vi "cursor window logic -- sygnal plot -- V3.vi"(4 "h. offset":dbl, 6 "CursIdx":i32, 7 "cursor window action":T3=enum."check", 8 "window":dbl=nan, 9 "center":dbl=nan, 10 "cursor window IN":refnum<vi>, 11 "cursor window init":T1={"left"=2378.60310421286, "right "=2421.6740576496672, "center"=2421.6740576496672, "window"=2421.6740576496672, "cursors"=[], "relative"=0, "absolute"=0, "fixed vertical offset"=2421.6740576496672, "vertical offset"=2421.6740576496672, "skew"=2421.6740576496672, "default window frac"=2421.6740576496672, "kind"=enum."skewed", "skew.left"=2421.6740576496672, "skew.right"=2421.6740576496672, "wing order"=enum."back", "Plot ref Syg"=refnum}) -> (2 "cursor window OUT":refnum<vi>, 3 "cursor window out":T1={"left"=2378.60310421286, "right "=2421.6740576496672, "center"=2421.6740576496672, "window"=2421.6740576496672, "cursors"=[], "relative"=0, "absolute"=0, "fixed vertical offset"=2421.6740576496672, "vertical offset"=2421.6740576496672, "skew"=2421.6740576496672, "default window frac"=2421.6740576496672, "kind"=enum."skewed", "skew.left"=2421.6740576496672, "skew.right"=2421.6740576496672, "wing order"=enum."back", "Plot ref Syg"=refnum})   [LabVIEW 2021]
uses:
  cursor window action.ctl
  cursor winow sygnal plot.ctl
  comparison control.ctl
  cursor window state.ctl
  stack action -- control.ctl
  cursor action.ctl
  2Dwindow-centerwin.ctl
  range multiplier action.ctl
  cursor sate.ctl
  replace cursor action stack.vi
  Q - not nan and gtr than zero - Real.vi
  Q - not nan -- real.vi
  array - smart min max.vi
  Q - not nan -- integer.vi
panel:
  in  "cursor window":T1={"left"=2378.60310421286, "right "=2421.6740576496672, "center"=2421.6740576496672, "window"=2421.6740576496672, "cursors"=[], "relative"=0, "absolute"=0, "fixed vertical offset"=2421.6740576496672, "vertical offset"=2421.6740576496672, "skew"=2421.6740576496672, "default window frac"=2421.6740576496672, "kind"=enum."skewed", "skew.left"=2421.6740576496672, "skew.right"=2421.6740576496672, "wing order"=enum."back", "Plot ref Syg"=refnum}
  out "Signal graph 2":waveform(dbl)[](graph)
  out "selector":T2
  out "result":bool
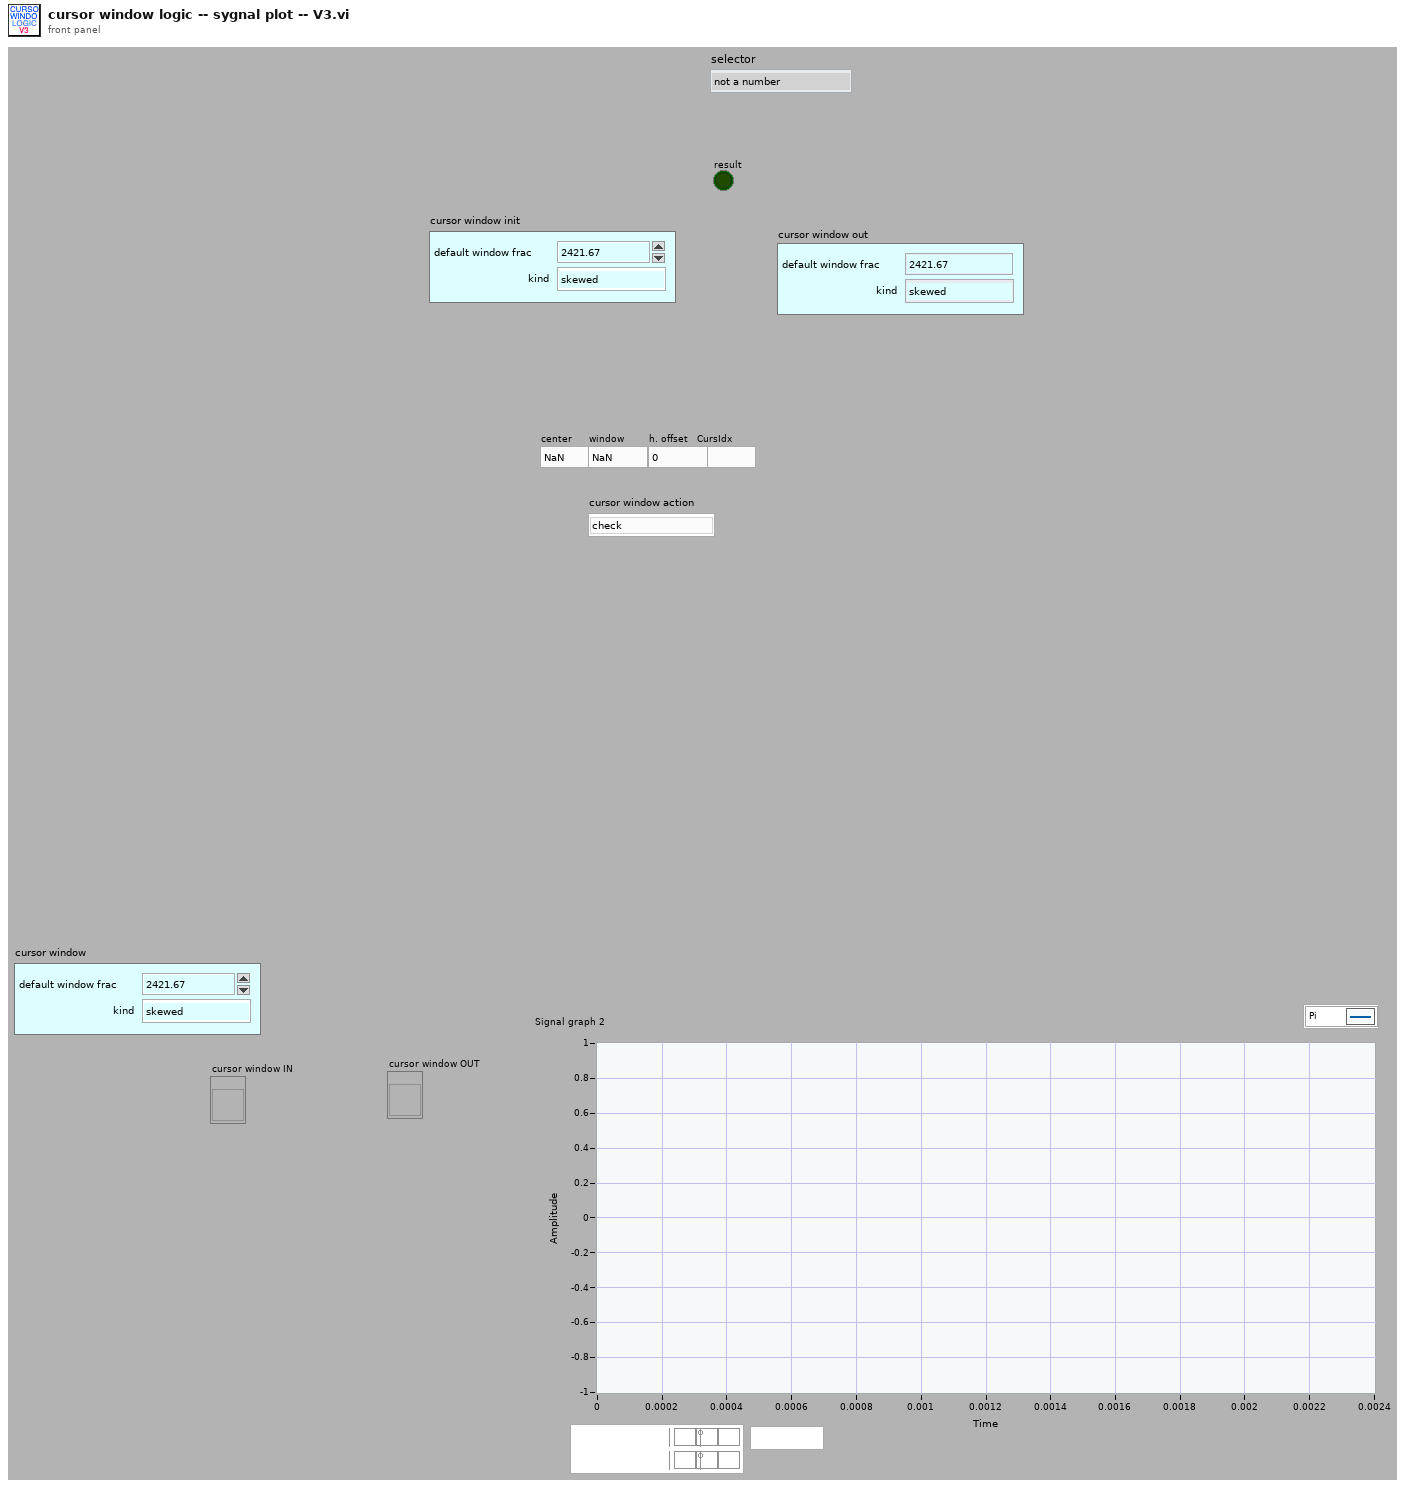
[diagram p1: front panel]
types:
  T1 = typedef "cursor winow sygnal plot.ctl" = cluster{"left":dbl, "right ":dbl, "center":dbl, "window":dbl, "cursors":i32[], "relative":i32, "absolute":i32, "fixed vertical offset":dbl, "vertical offset":dbl, "skew":dbl, "default window frac":dbl, "kind":enum16{"symmetric", "skewed", "fancy"}, "skew.left":dbl, "skew.right":dbl, "wing order":enum16{"forw", "back"}, "Plot ref Syg":refnum<vi>}
  T2 = typedef "comparison control.ctl" = enum16{"not a number", "above", "in range", "below"}
  T3 = typedef "cursor window action.ctl" = enum16{"balance", "h. offset change", "cursor moves", "change center", "change window", "init", "check", "reset", "set y to middle", "idle", "-write all Y", "-write left.X", "-write center.X", "-write right.X", "-write all X", "-change center", "-change window", "-change skew", "-read cursor 2", "-read cursor 1", "-read cursor 0", "-read all cursors", "-reset", "-read plot scale", "-set y to middle", "-Q: center.Y is visible", "-Q: window is visible", "-parse center.Y", "-right left from center", "-left move", "-right move", "-set center.Y", "-empty", "-set cursors to default", "-check", "-write center.Y", "-copy cursor 1", "-copy cursor 0", "-copy cursor 2", "move right", "move left", "shrink", "broaden", "skew up", "skew down", "-write plot scale", "zoom X", "change cen&win", "zoom to all data", "color--red", "color--green", "color--yellow", "read", "zoom out", "zoom in", "slide right", "slide left", "set range aspect ratio to 1", "move to window range", "--move to window range"}
  T4 = typedef "cursor window state.ctl" = cluster{"scale.y.halfwidth":dbl, "scale.y.center":dbl, "scale.x.halfwidth":dbl, "scale.x.center":dbl, "cursor":i32, "skew":dbl, "scale.y.max":dbl, "scale.x.range":dbl, "scale.y.min":dbl, "scale.y.range":dbl, "scale.x.min":dbl, "scale.x.max":dbl, "center.Y":dbl, "center.X":dbl, "left.Y":dbl, "left.X":dbl, "right.X":dbl, "right.Y":dbl}
  T5 = typedef "stack action -- control.ctl" = enum16{"push", "pop", "check", "init"}
  T6 = cluster{"center":dbl, "window":dbl, "h.offset":dbl, "cursor window":T1}
  T7 = typedef "cursor action.ctl" = enum16{"range", "read", "write", "check", "zoom out", "smart zoom out", "zoom to aspect ratio 1", "zoom to win", "zoom out 20%", "zoom in 20%", "-empty", "smart zoom out&aspect", "move range left 20%", "move range right 20%", "move range up 20%", "move range down 20%", "zoom to X win", "zoom to Y win", "zoom out X", "zoom out Y", "zoom in X", "zoom in Y", "check plot scale", "set plot color", "set Xlabel", "set Ylabel", "set cursor color", "setlength", "empty", "hide plot", "unhide plot", "checklngth", "extend +1 if short", "extend +n if short"}
  T8 = typedef "2Dwindow-centerwin.ctl" = cluster{"window y":dbl, "center x":dbl, "center y":dbl, "window x":dbl}
  T9 = typedef "range multiplier action.ctl" = enum16{"shift", "zoom", "check"}
  T10 = typedef "2Dwindow-bounds.ctl" = cluster{"min y":dbl, "max x":dbl, "min x":dbl, "max y":dbl}
  T11 = typedef "cursor sate.ctl" = enum16{"normal", "alert", "fuzzy", "interesting", "boring", "colored"}
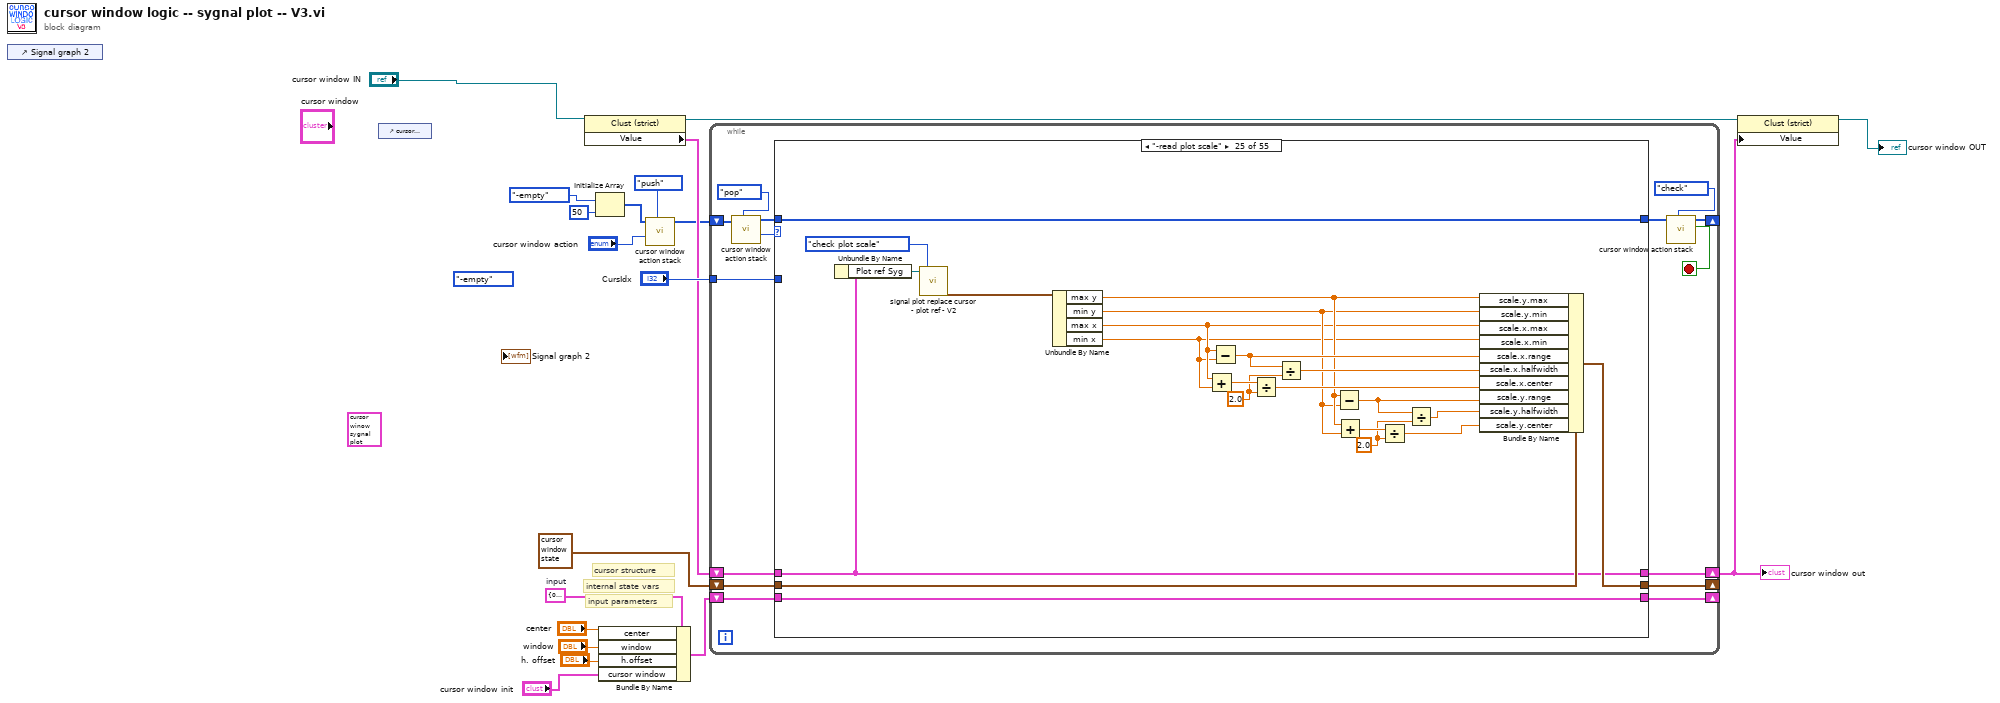
[diagram p0: block diagram]
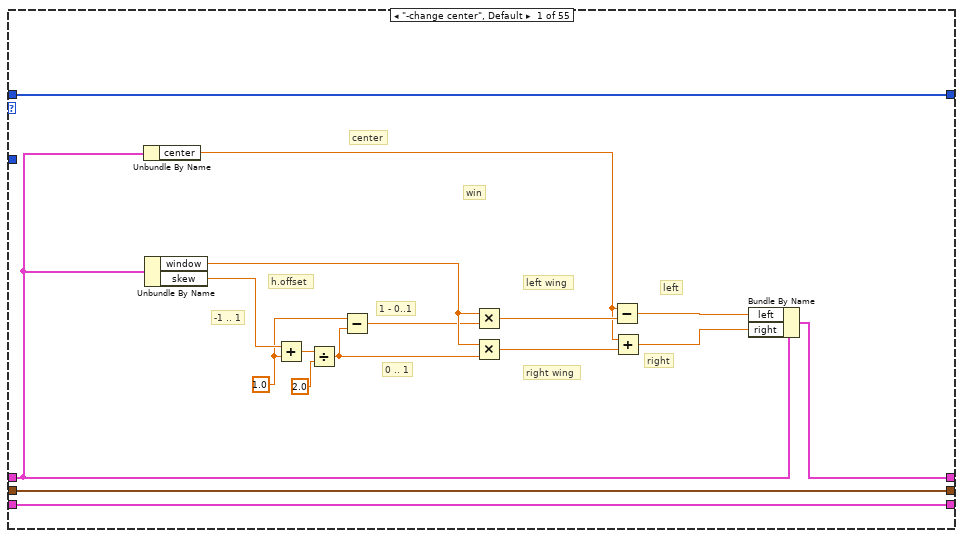
[diagram p2: hidden frame]
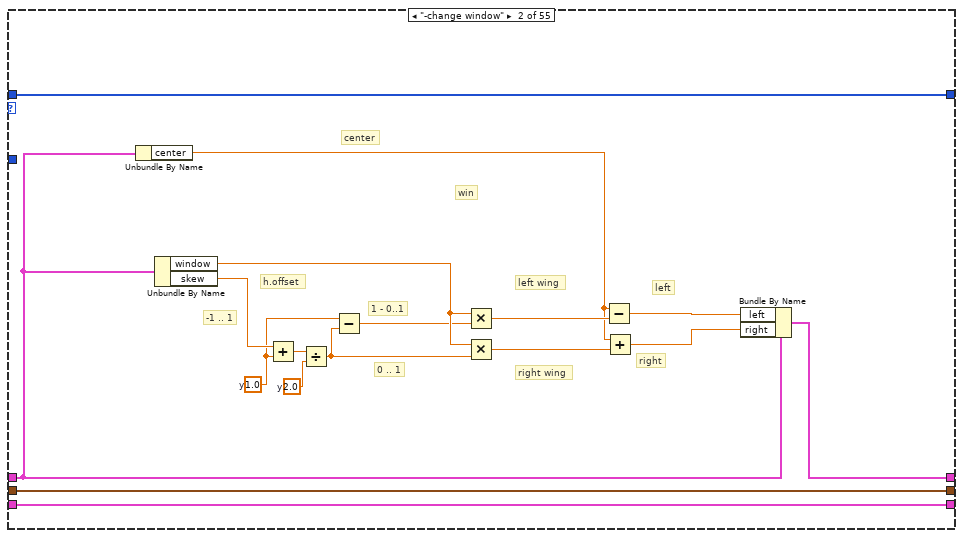
[diagram p3: hidden frame]
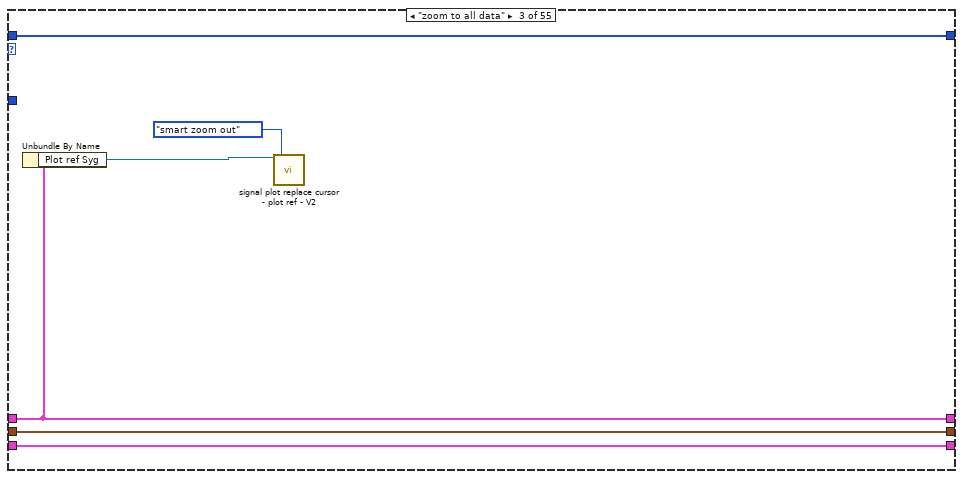
[diagram p4: hidden frame]
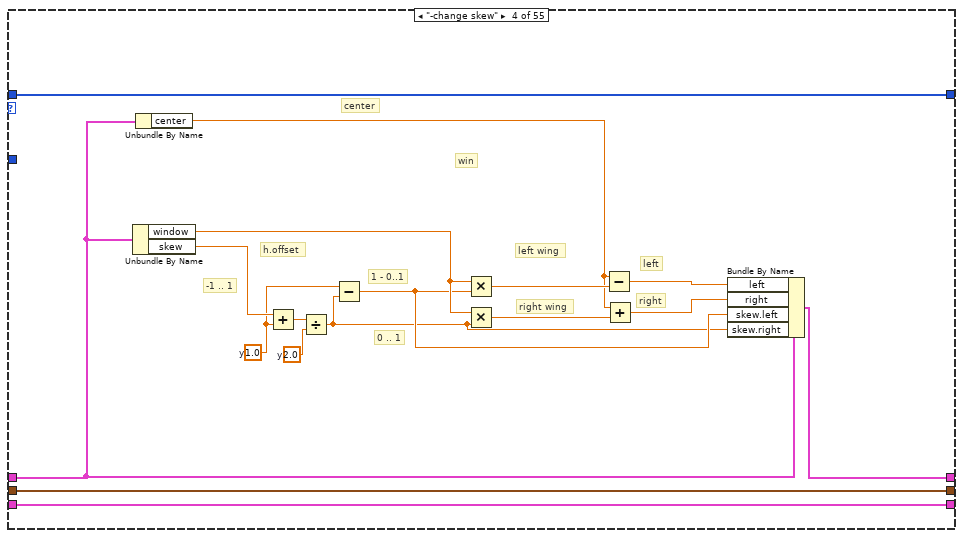
[diagram p5: hidden frame]
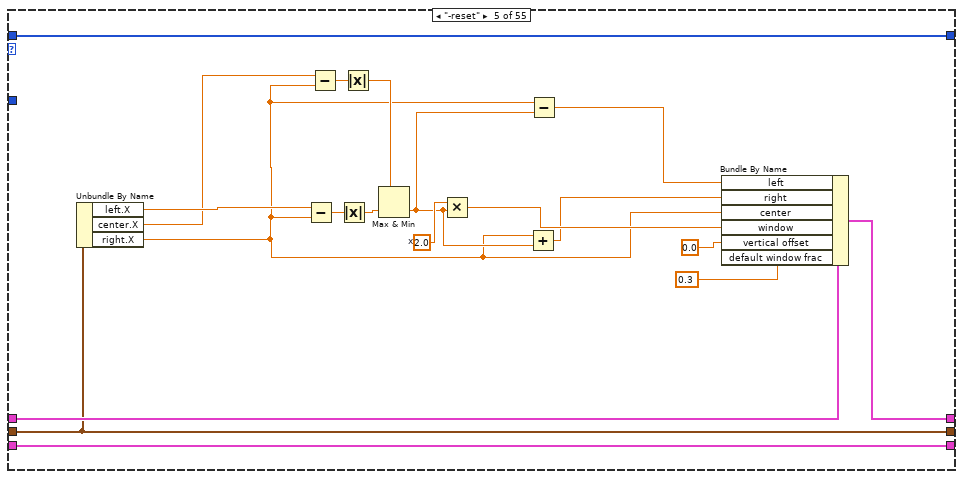
[diagram p6: hidden frame]
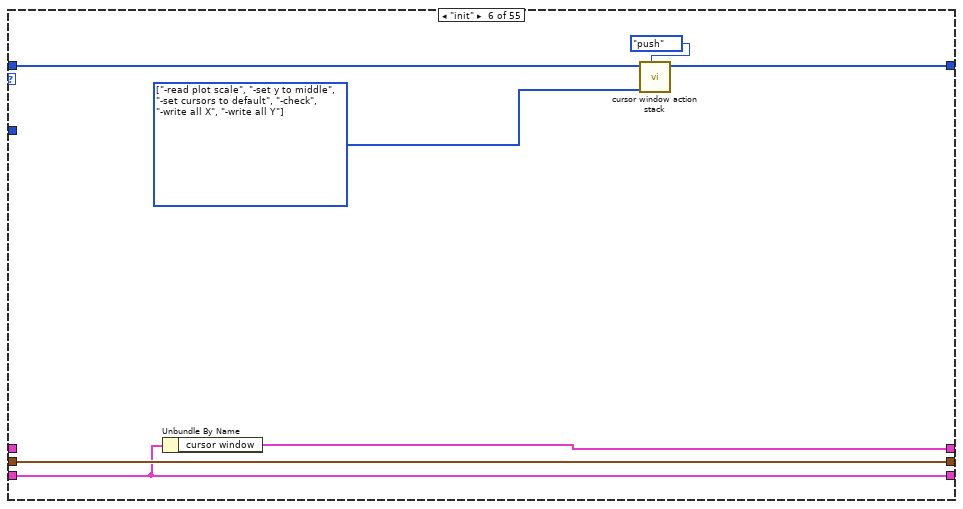
[diagram p7: hidden frame]
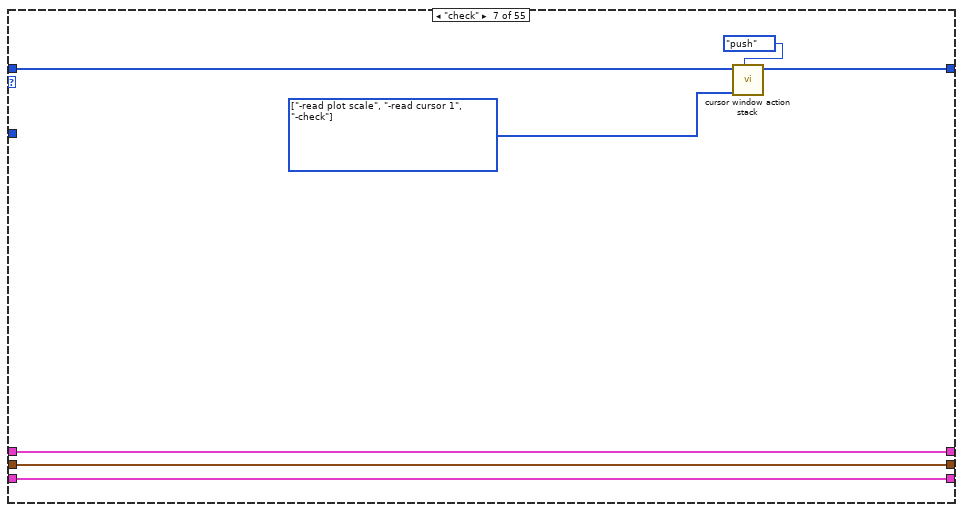
[diagram p8: hidden frame]
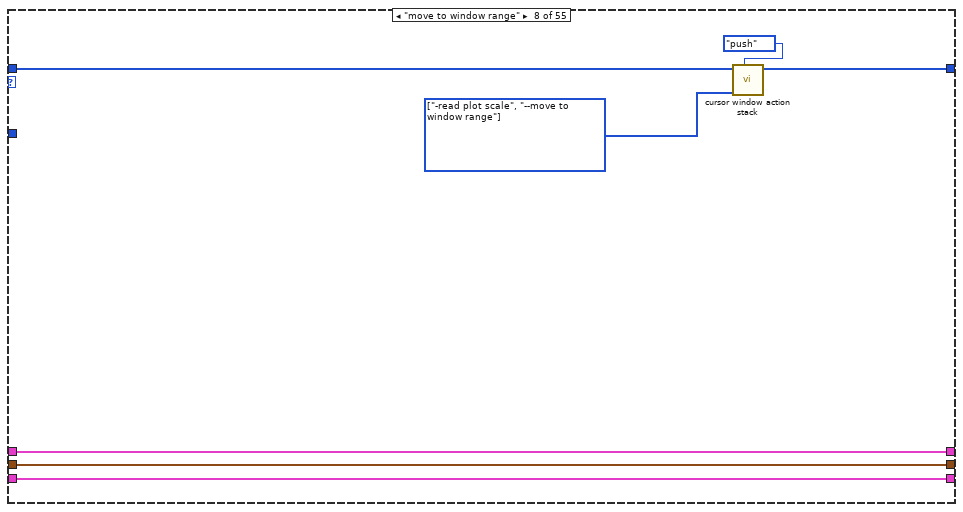
[diagram p9: hidden frame]
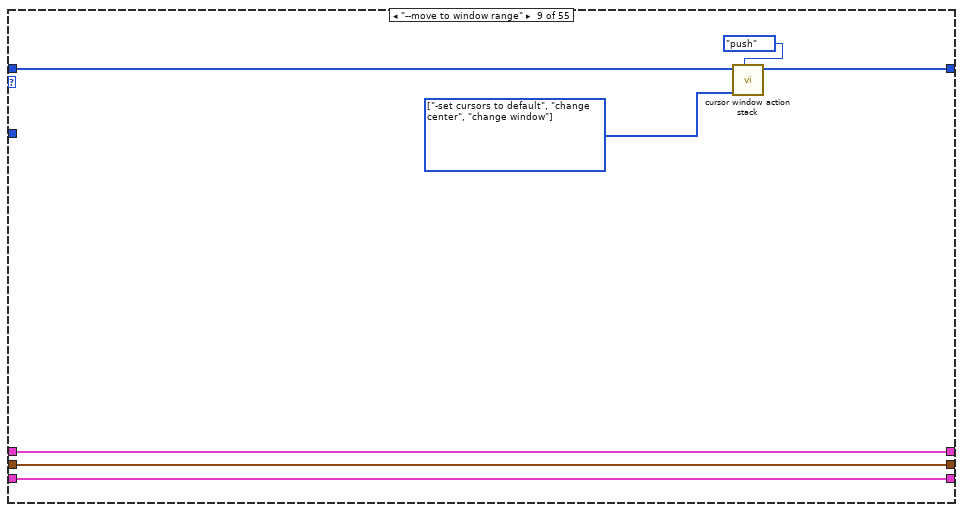
[diagram p10: hidden frame]
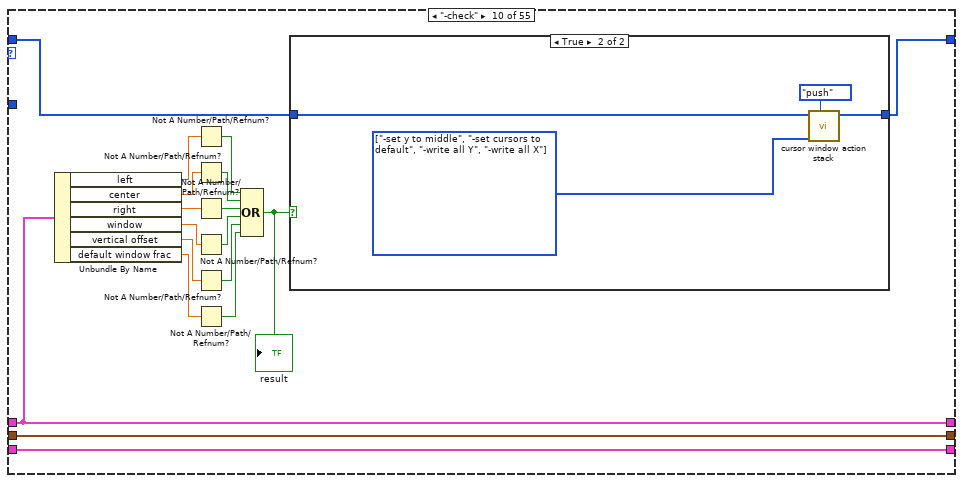
[diagram p11: hidden frame]
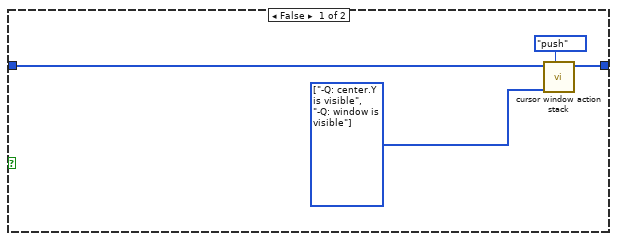
[diagram p12: hidden frame]
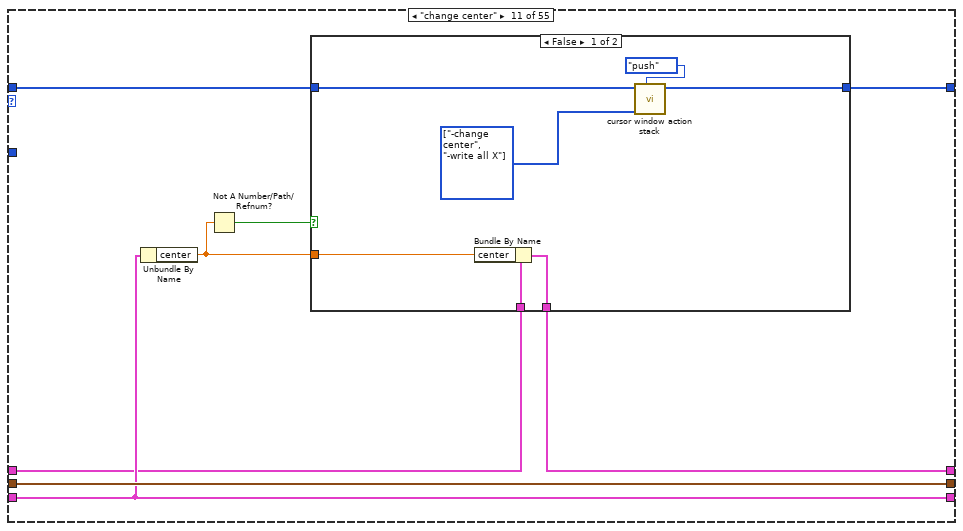
[diagram p13: hidden frame]
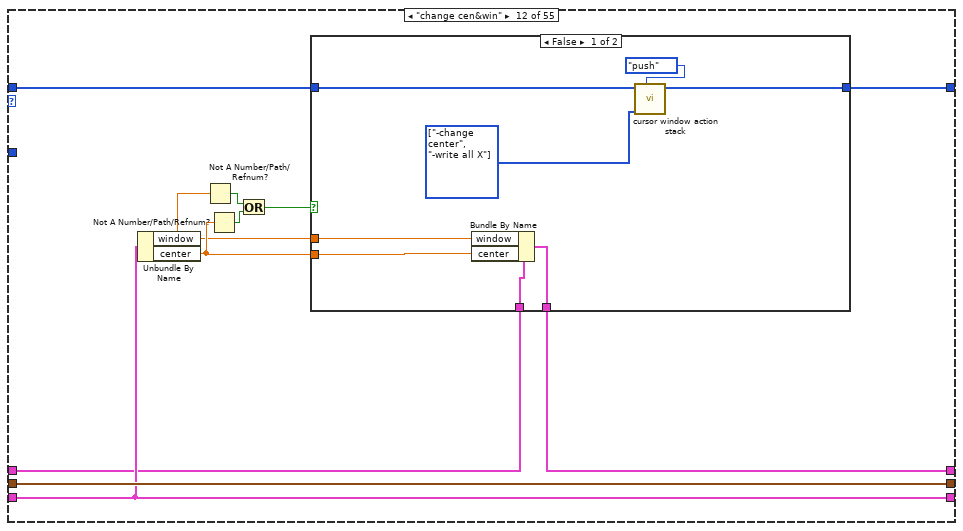
[diagram p15: hidden frame]
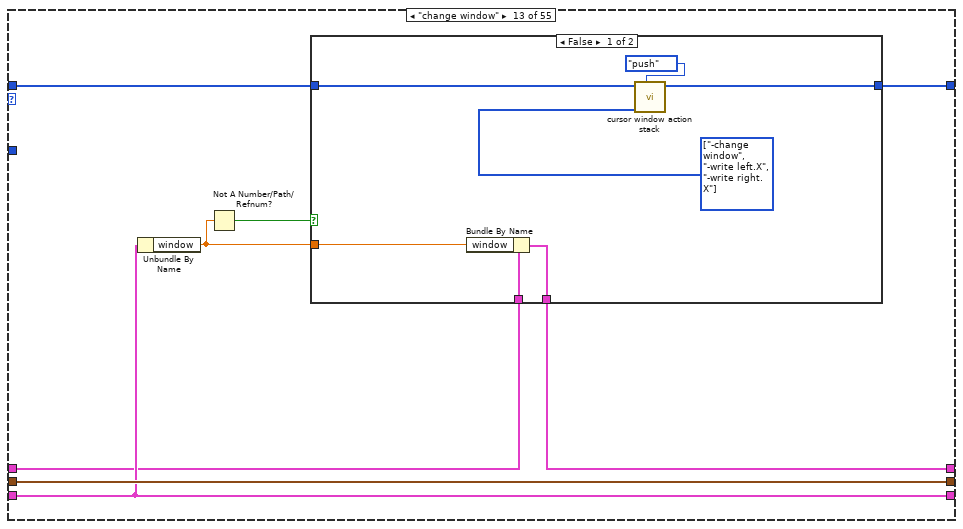
[diagram p17: hidden frame]
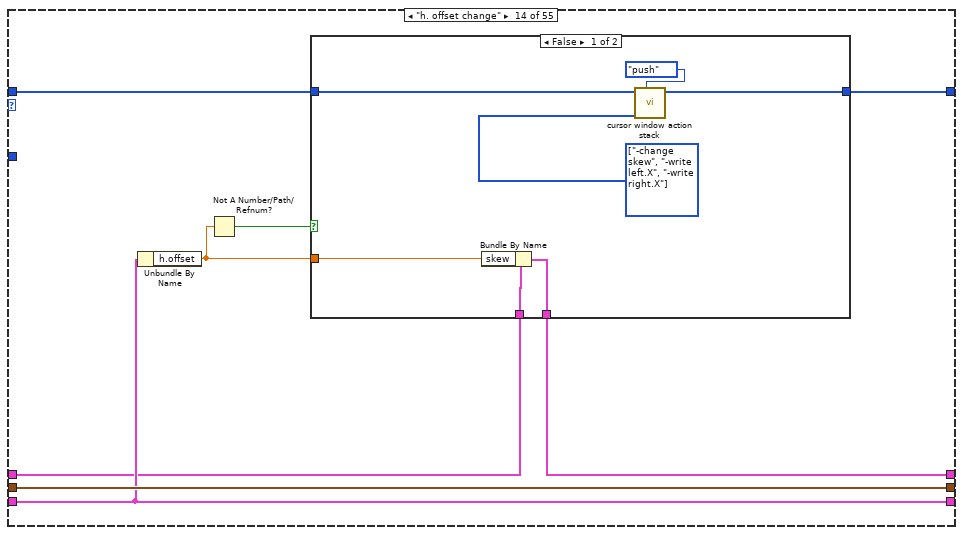
[diagram p19: hidden frame]
diagram:
  (unwired) T1 {"left"=2378.60310421286, "right "=2421.6740576496672, "center"=2421.6740576496672, "window"=2421.6740576496672, "cursors"=[], "relative"=0, "absolute"=0, "fixed vertical offset"=2421.6740576496672, "vertical offset"=2421.6740576496672, "skew"=2421.6740576496672, "default window frac"=2421.6740576496672, "kind"=enum."skewed", "skew.left"=2421.6740576496672, "skew.right"=2421.6740576496672, "wing order"=enum."back", "Plot ref Syg"=refnum} ("cursor window")
  (unwired) cursor_window_action."-empty" ("cursor window action")
  w18 = T6 {"center"=0.0, "window"=0.0, "h.offset"=0.0, "cursor window"={"left"=2378.60310421286, "right "=2421.6740576496672, "center"=2421.6740576496672, "window"=2421.6740576496672, "cursors"=[], "relative"=0, "absolute"=0, "fixed vertical offset"=2421.6740576496672, "vertical offset"=2421.6740576496672, "skew"=2421.6740576496672, "default window frac"=2421.6740576496672, "kind"=enum."skewed", "skew.left"=2421.6740576496672, "skew.right"=2421.6740576496672, "wing order"=enum."back", "Plot ref Syg"=refnum}}  # input
  # "input parameters"
  # "internal state vars"
  # "cursor structure"
  n1 = control-ref of="Signal graph 2"() -> ()  [unwired: 1 out]
  n2 = control-ref of="cursor window"() -> ()  [unwired: 1 out]
  n3 = property class="Clust (strict)"(reference="cursor window IN") -> (reference out=w19:refnum<vi>, "Value"=w12:T1)  [unwired: 1 in, 1 out]
  n4 = Initialize Array(cursor_window_action."-empty" ("cursor window action"), 50 ("dimension size")) -> (w7:T3[])
  n5 = Bundle By Name(cluster=w18, "center"="center", "window"="window", "h.offset"="h. offset", "cursor window"="cursor window init") -> (w14:T6)
  n6 = call "cursor window action stack.vi"("stack action"=stack_action_--_control."push", "cursor window action"="cursor window action", "command stack"=w7) -> ("command stack out"=w6:T3[])  [unwired: 6 in, 2 out]
  n7 = while {
    shift-right: [w27] -> _
    shift-left: w6 -> [w33]
    shift-right: [w20] -> w11
    shift-left: w12 -> [w34]
    shift-right: [w24] -> _
    shift-left: w14 -> [w25]
    shift-right: [w22] -> _
    shift-left: T4 {"scale.y.halfwidth"=nan, "scale.y.center"=nan, "scale.x.halfwidth"=nan, "scale.x.center"=nan, "cursor"=0, "skew"=nan, "scale.y.max"=nan, "scale.x.range"=nan, "scale.y.min"=nan, "scale.y.range"=nan, "scale.x.min"=nan, "scale.x.max"=nan, "center.Y"=nan, "center.X"=nan, "left.Y"=nan, "left.X"=nan, "right.X"=nan, "right.Y"=nan} ("state variables") -> [w23]
    tunnel: "CursIdx" -> [w21]
    stop <- w26 stop-if-true
    n8 = call "cursor window action stack.vi"("stack action"=stack_action_--_control."pop", "command stack"=w33) -> ("cursor window action out"=w32:T3, "command stack out"=w30:T3[])  [unwired: 7 in, 1 out]
    n9 = case shown="\"-read plot scale\"" w32 {
      tunnel: w34 -> [w36 w53 w71 w78 w100 _ w118 w125 w132 w142 w166 w187 w204 w221 w237 w244 w261 w295 w330 w369 w401 w405 w412 w431 w445 w471 w486 w492 w498 w504 w510 w516 w523 w547 w553 w573 w579 w592 w613 w652 w686 w726 w747 w767 w787 w808 w822 w839 w858 w871 w880 w903 w907 w920 w934]
      tunnel: [w40 w57 w74 w82 w99 w112 w121 w128 w135 w139 w171 w191 w209 w226 w240 w247 w258 w292 w332 w370 w402 w403 w421 w437 w456 w472 w487 w493 w499 w505 w511 w517 w521 w548 w561 w574 w588 w596 w617 w650 w688 w743 w763 w783 w803 w821 w836 w853 w867 w879 w901 w905 w919 w933 w947] -> w28
      tunnel: w30 -> [w40 w57 w74 w82 w99 w113 w122 w129 w136 w140 w170 w190 w208 w225 w241 w248 w258 w292 w332 w357 w402 w403 w421 w437 w456 w472 w487 w493 w499 w505 w511 w517 w522 w549 w562 w575 w589 w597 w618 w650 w689 w743 w763 w783 w803 w821 w836 w853 w867 w879 w901 w905 w919 w933 w947]
      tunnel: w25 -> [w37 w54 w72 w79 w98 w116 w119 w126 w133 w143 w169 w189 w207 w224 w243 w250 w260 w294 w331 w362 w399 w406 w420 w436 w459 w473 w488 w494 w500 w506 w512 w518 w529 w543 w559 w569 w586 w593 w614 w668 w693 w728 w749 w769 w789 w810 w828 w846 w860 w873 w882 w904 w909 w923 w937]
      tunnel: [w37 w54 w72 w79 w98 w116 w119 w126 w133 w143 w169 w189 w207 w224 w243 w250 w260 w294 w331 w362 w399 w406 w420 w436 w459 w473 w488 w494 w500 w506 w512 w518 w529 w543 w559 w569 w586 w593 w614 w668 w693 w728 w749 w769 w789 w810 w828 w846 w860 w873 w882 w904 w909 w923 w937] -> w24
      tunnel: w23 -> [w39 w56 w73 w81 w97 w117 w120 w127 w134 w144 w172 w192 w210 w227 w242 w249 w259 w293 w336 w363 w400 w408 w417 w435 w458 w470 w485 w491 w497 w503 w509 w515 w525 w544 w560 w570 w587 w594 w615 w656 w692 w729 w750 w770 w790 w807 w829 w847 w861 w870 w890 w902 w913 w927 w941]
      tunnel: [w39 w56 w73 w81 w97 w117 w120 w127 w134 w144 w172 w192 w210 w227 w242 w249 w259 w293 w335 w363 w400 w408 w416 w435 w457 w470 w485 w491 w497 w503 w509 w515 w524 w544 w560 w570 w587 w594 w615 w659 w692 w729 w750 w770 w790 w807 w829 w847 w861 w870 w889 w902 w912 w926 w940] -> w22
      tunnel: w21 -> [_ _ _ _ _ _ _ _ _ _ _ _ _ _ _ _ _ _ _ w360 _ _ _ _ _ _ _ _ _ _ _ _ _ _ _ _ _ _ _ _ _ _ _ _ _ _ _ _ _ _ _ _ _ _ _]
      tunnel: [w35 w52 w71 w77 w93 w111 w118 w125 w132 w142 w165 w186 w203 w220 w237 w244 w251 w285 w330 w361 w401 w404 w411 w427 w445 w471 w486 w492 w498 w504 w510 w516 w523 w546 w552 w572 w578 w595 w616 w648 w685 w726 w747 w767 w787 w808 w822 w839 w858 w871 w880 w903 w907 w920 w934] -> w20
      frame "-change center", Default {
        w45 = 1.0 ("y")
        # "1 - 0..1"
        # "right"
        # "left"
        # "win"
        # "h.offset"
        # "center"
        # "left wing"
        # "right wing"
        # "0 .. 1"
        # "-1 .. 1"
        n10 = Unbundle By Name(w36) -> ("center"=w38:dbl)
        n11 = Unbundle By Name(w36) -> ("window"=w50:dbl, "skew"=w51:dbl)
        n12 = Add(x=w51, y=w45) -> (x+y=w46:dbl)
        n13 = Divide(x=w46, y=2.0) -> (x/y=w42:dbl)
        n14 = Subtract(x=w45, y=w42) -> (x-y=w41:dbl)
        n15 = Multiply(x=w50, y=w41) -> (x*y=w44:dbl)
        n16 = Multiply(x=w50, y=w42) -> (x*y=w43:dbl)
        n17 = Subtract(x=w38, y=w44) -> (x-y=w49:dbl)
        n18 = Add(x=w38, y=w43) -> (x+y=w48:dbl)
        n19 = Bundle By Name(cluster=w36, "left"=w49, "right"=w48) -> (w35:T1)
      }
      frame "-change window" {
        w62 = 1.0  # y
        w64 = 2.0  # y
        # "1 - 0..1"
        # "right"
        # "left"
        # "win"
        # "h.offset"
        # "center"
        # "left wing"
        # "right wing"
        # "0 .. 1"
        # "-1 .. 1"
        n20 = Unbundle By Name(w53) -> ("center"=w55:dbl)
        n21 = Unbundle By Name(w53) -> ("window"=w67:dbl, "skew"=w68:dbl)
        n22 = Add(x=w68, y=w62) -> (x+y=w63:dbl)
        n23 = Divide(x=w63, y=w64) -> (x/y=w59:dbl)
        n24 = Subtract(x=w62, y=w59) -> (x-y=w58:dbl)
        n25 = Multiply(x=w67, y=w58) -> (x*y=w61:dbl)
        n26 = Multiply(x=w67, y=w59) -> (x*y=w60:dbl)
        n27 = Subtract(x=w55, y=w61) -> (x-y=w66:dbl)
        n28 = Add(x=w55, y=w60) -> (x+y=w65:dbl)
        n29 = Bundle By Name(cluster=w53, "left"=w66, "right"=w65) -> (w52:T1)
      }
      frame "zoom to all data" {
        n30 = Unbundle By Name(w71) -> ("Plot ref Syg"=w69:refnum<vi>)
        n31 = call "signal plot replace cursor - plot ref - V2.vi"("Signal graph IN"=w69, "cursor action"=cursor_action."smart zoom out") -> ()  [unwired: 14 in, 4 out]
      }
      frame "-change skew" {
        w85 = 1.0  # y
        w87 = 2.0  # y
        # "1 - 0..1"
        # "right"
        # "left"
        # "win"
        # "h.offset"
        # "center"
        # "left wing"
        # "right wing"
        # "0 .. 1"
        # "-1 .. 1"
        n32 = Unbundle By Name(w78) -> ("window"=w90:dbl, "skew"=w91:dbl)
        n33 = Unbundle By Name(w78) -> ("center"=w80:dbl)
        n34 = Add(x=w91, y=w85) -> (x+y=w86:dbl)
        n35 = Divide(x=w86, y=w87) -> (x/y=w75:dbl)
        n36 = Subtract(x=w85, y=w75) -> (x-y=w76:dbl)
        n37 = Multiply(x=w90, y=w76) -> (x*y=w84:dbl)
        n38 = Multiply(x=w90, y=w75) -> (x*y=w83:dbl)
        n39 = Subtract(x=w80, y=w84) -> (x-y=w89:dbl)
        n40 = Add(x=w80, y=w83) -> (x+y=w88:dbl)
        n41 = Bundle By Name(cluster=w78, "left"=w89, "right"=w88, "skew.left"=w76, "skew.right"=w75) -> (w77:T1)
      }
      frame "-reset" {
        w106 = 2.0  # x
        n42 = Unbundle By Name(w97) -> ("left.X"=w96:dbl, "center.X"=w94:dbl, "right.X"=w95:dbl)
        n43 = Subtract(x=w96, y=w95) -> (x-y=w109:dbl)
        n44 = Subtract(x=w94, y=w95) -> (x-y=w110:dbl)
        n45 = Absolute Value(x=w109) -> (abs(x)=w107:dbl)
        n46 = Absolute Value(x=w110) -> (abs(x)=w108:dbl)
        n47 = Max & Min(x=w108, y=w107) -> (min(x,y)=w104:dbl)  [unwired: 1 out]
        n48 = Multiply(x=w106, y=w104) -> (x*y=w105:dbl)
        n49 = Add(x=w95, y=w104) -> (x+y=w102:dbl)
        n50 = Subtract(x=w95, y=w104) -> (x-y=w103:dbl)
        n51 = Bundle By Name(cluster=w100, "left"=w103, "right"=w102, "center"=w95, "window"=w105, "vertical offset"=0.0, "default window frac"=0.3) -> (w93:T1)
      }
      frame "init" {
        w114 = T3[] [enum."-read plot scale", enum."-set y to middle", enum."-set cursors to default", enum."-check", enum."-write all X", enum."-write all Y"] items=["balance", "h. offset change", "cursor moves", "change center", "change window", "init", "check", "reset", "set y to middle", "idle", "-write all Y", "-write left.X", "-write center.X", "-write right.X", "-write all X", "-change center", "-change window", "-change skew", "-read cursor 2", "-read cursor 1", "-read cursor 0", "-read all cursors", "-reset", "-read plot scale", "-set y to middle", "-Q: center.Y is visible", "-Q: window is visible", "-parse center.Y", "-right left from center", "-left move", "-right move", "-set center.Y", "-empty", "-set cursors to default", "-check", "-write center.Y", "-copy cursor 1", "-copy cursor 0", "-copy cursor 2", "move right", "move left", "shrink", "broaden", "skew up", "skew down", "-write plot scale", "zoom X", "change cen&win", "zoom to all data", "color--red", "color--green", "color--yellow", "read", "zoom out", "zoom in", "slide right", "slide left", "set range aspect ratio to 1", "move to window range", "--move to window range"]
        n52 = Unbundle By Name(w116) -> ("cursor window"=w111:T1)
        n53 = call "cursor window action stack.vi"("stack action"=stack_action_--_control."push", "action list"=w114, "command stack"=w113) -> ("command stack out"=w112:T3[])  [unwired: 6 in, 2 out]
      }
      frame "check" {
        w123 = T3[] [enum."-read plot scale", enum."-read cursor 1", enum."-check"] items=["balance", "h. offset change", "cursor moves", "change center", "change window", "init", "check", "reset", "set y to middle", "idle", "-write all Y", "-write left.X", "-write center.X", "-write right.X", "-write all X", "-change center", "-change window", "-change skew", "-read cursor 2", "-read cursor 1", "-read cursor 0", "-read all cursors", "-reset", "-read plot scale", "-set y to middle", "-Q: center.Y is visible", "-Q: window is visible", "-parse center.Y", "-right left from center", "-left move", "-right move", "-set center.Y", "-empty", "-set cursors to default", "-check", "-write center.Y", "-copy cursor 1", "-copy cursor 0", "-copy cursor 2", "move right", "move left", "shrink", "broaden", "skew up", "skew down", "-write plot scale", "zoom X", "change cen&win", "zoom to all data", "color--red", "color--green", "color--yellow", "read", "zoom out", "zoom in", "slide right", "slide left", "set range aspect ratio to 1", "move to window range", "--move to window range"]
        n54 = call "cursor window action stack.vi"("stack action"=stack_action_--_control."push", "action list"=w123, "command stack"=w122) -> ("command stack out"=w121:T3[])  [unwired: 6 in, 2 out]
      }
      frame "move to window range" {
        w130 = T3[] [enum."-read plot scale", enum."--move to window range"] items=["balance", "h. offset change", "cursor moves", "change center", "change window", "init", "check", "reset", "set y to middle", "idle", "-write all Y", "-write left.X", "-write center.X", "-write right.X", "-write all X", "-change center", "-change window", "-change skew", "-read cursor 2", "-read cursor 1", "-read cursor 0", "-read all cursors", "-reset", "-read plot scale", "-set y to middle", "-Q: center.Y is visible", "-Q: window is visible", "-parse center.Y", "-right left from center", "-left move", "-right move", "-set center.Y", "-empty", "-set cursors to default", "-check", "-write center.Y", "-copy cursor 1", "-copy cursor 0", "-copy cursor 2", "move right", "move left", "shrink", "broaden", "skew up", "skew down", "-write plot scale", "zoom X", "change cen&win", "zoom to all data", "color--red", "color--green", "color--yellow", "read", "zoom out", "zoom in", "slide right", "slide left", "set range aspect ratio to 1", "move to window range", "--move to window range"]
        n55 = call "cursor window action stack.vi"("stack action"=stack_action_--_control."push", "action list"=w130, "command stack"=w129) -> ("command stack out"=w128:T3[])  [unwired: 6 in, 2 out]
      }
      frame "--move to window range" {
        w137 = T3[] [enum."-set cursors to default", enum."change center", enum."change window"] items=["balance", "h. offset change", "cursor moves", "change center", "change window", "init", "check", "reset", "set y to middle", "idle", "-write all Y", "-write left.X", "-write center.X", "-write right.X", "-write all X", "-change center", "-change window", "-change skew", "-read cursor 2", "-read cursor 1", "-read cursor 0", "-read all cursors", "-reset", "-read plot scale", "-set y to middle", "-Q: center.Y is visible", "-Q: window is visible", "-parse center.Y", "-right left from center", "-left move", "-right move", "-set center.Y", "-empty", "-set cursors to default", "-check", "-write center.Y", "-copy cursor 1", "-copy cursor 0", "-copy cursor 2", "move right", "move left", "shrink", "broaden", "skew up", "skew down", "-write plot scale", "zoom X", "change cen&win", "zoom to all data", "color--red", "color--green", "color--yellow", "read", "zoom out", "zoom in", "slide right", "slide left", "set range aspect ratio to 1", "move to window range", "--move to window range"]
        n56 = call "cursor window action stack.vi"("stack action"=stack_action_--_control."push", "action list"=w137, "command stack"=w136) -> ("command stack out"=w135:T3[])  [unwired: 6 in, 2 out]
      }
      frame "-check" {
        n57 = Unbundle By Name(w142) -> ("left"=w154:dbl, "center"=w153:dbl, "right"=w155:dbl, "window"=w156:dbl, "vertical offset"=w148:dbl, "default window frac"=w147:dbl)
        n58 = Not A Number/Path/Refnum?(number/path/refnum=w154) -> (NaN/Path/Refnum?=w152:bool)
        n59 = Not A Number/Path/Refnum?(number/path/refnum=w153) -> (NaN/Path/Refnum?=w151:bool)
        n60 = Not A Number/Path/Refnum?(number/path/refnum=w155) -> (NaN/Path/Refnum?=w150:bool)
        n61 = Not A Number/Path/Refnum?(number/path/refnum=w156) -> (NaN/Path/Refnum?=w149:bool)
        n62 = Not A Number/Path/Refnum?(number/path/refnum=w148) -> (NaN/Path/Refnum?=w145:bool)
        n63 = Not A Number/Path/Refnum?(number/path/refnum=w147) -> (NaN/Path/Refnum?=w146:bool)
        n64 = Compound Arithmetic op=OR(w152, w151, w150, w149, w145, w146) -> (w141:bool)
        "result" <- w141
        n65 = case shown="True" w141 {
          tunnel: w140 -> [w158 w162]
          tunnel: [w157 w161] -> w139
          frame False {
            w159 = T3[] [enum."-Q: center.Y is visible", enum."-Q: window is visible"] items=["balance", "h. offset change", "cursor moves", "change center", "change window", "init", "check", "reset", "set y to middle", "idle", "-write all Y", "-write left.X", "-write center.X", "-write right.X", "-write all X", "-change center", "-change window", "-change skew", "-read cursor 2", "-read cursor 1", "-read cursor 0", "-read all cursors", "-reset", "-read plot scale", "-set y to middle", "-Q: center.Y is visible", "-Q: window is visible", "-parse center.Y", "-right left from center", "-left move", "-right move", "-set center.Y", "-empty", "-set cursors to default", "-check", "-write center.Y", "-copy cursor 1", "-copy cursor 0", "-copy cursor 2", "move right", "move left", "shrink", "broaden", "skew up", "skew down", "-write plot scale", "zoom X", "change cen&win", "zoom to all data", "color--red", "color--green", "color--yellow", "read", "zoom out", "zoom in", "slide right", "slide left", "set range aspect ratio to 1", "move to window range", "--move to window range"]
            n66 = call "cursor window action stack.vi"("stack action"=stack_action_--_control."push", "action list"=w159, "command stack"=w158) -> ("command stack out"=w157:T3[])  [unwired: 6 in, 2 out]
          }
          frame True {
            w163 = T3[] [enum."-set y to middle", enum."-set cursors to default", enum."-write all Y", enum."-write all X"] items=["balance", "h. offset change", "cursor moves", "change center", "change window", "init", "check", "reset", "set y to middle", "idle", "-write all Y", "-write left.X", "-write center.X", "-write right.X", "-write all X", "-change center", "-change window", "-change skew", "-read cursor 2", "-read cursor 1", "-read cursor 0", "-read all cursors", "-reset", "-read plot scale", "-set y to middle", "-Q: center.Y is visible", "-Q: window is visible", "-parse center.Y", "-right left from center", "-left move", "-right move", "-set center.Y", "-empty", "-set cursors to default", "-check", "-write center.Y", "-copy cursor 1", "-copy cursor 0", "-copy cursor 2", "move right", "move left", "shrink", "broaden", "skew up", "skew down", "-write plot scale", "zoom X", "change cen&win", "zoom to all data", "color--red", "color--green", "color--yellow", "read", "zoom out", "zoom in", "slide right", "slide left", "set range aspect ratio to 1", "move to window range", "--move to window range"]
            n67 = call "cursor window action stack.vi"("stack action"=stack_action_--_control."push", "action list"=w163, "command stack"=w162) -> ("command stack out"=w161:T3[])  [unwired: 6 in, 2 out]
          }
        }
      }
      frame "change center" {
        n68 = Unbundle By Name(w169) -> ("center"=w167:dbl)
        n69 = Not A Number/Path/Refnum?(number/path/refnum=w167) -> (NaN/Path/Refnum?=w168:bool)
        n70 = case shown="False" w168 {
          tunnel: [w179 w180] -> w171
          tunnel: w170 -> [w178 w180]
          tunnel: w166 -> [w175 w181]
          tunnel: w167 -> [w174 _]
          tunnel: [w173 w181] -> w165
          frame False {
            w176 = T3[] [enum."-change center", enum."-write all X"] items=["balance", "h. offset change", "cursor moves", "change center", "change window", "init", "check", "reset", "set y to middle", "idle", "-write all Y", "-write left.X", "-write center.X", "-write right.X", "-write all X", "-change center", "-change window", "-change skew", "-read cursor 2", "-read cursor 1", "-read cursor 0", "-read all cursors", "-reset", "-read plot scale", "-set y to middle", "-Q: center.Y is visible", "-Q: window is visible", "-parse center.Y", "-right left from center", "-left move", "-right move", "-set center.Y", "-empty", "-set cursors to default", "-check", "-write center.Y", "-copy cursor 1", "-copy cursor 0", "-copy cursor 2", "move right", "move left", "shrink", "broaden", "skew up", "skew down", "-write plot scale", "zoom X", "change cen&win", "zoom to all data", "color--red", "color--green", "color--yellow", "read", "zoom out", "zoom in", "slide right", "slide left", "set range aspect ratio to 1", "move to window range", "--move to window range"]
            n71 = Bundle By Name(cluster=w175, "center"=w174) -> (w173:T1)
            n72 = call "cursor window action stack.vi"("stack action"=stack_action_--_control."push", "action list"=w176, "command stack"=w178) -> ("command stack out"=w179:T3[])  [unwired: 6 in, 2 out]
          }
          frame True {
          }
        }
      }
      frame "change cen&win" {
        n73 = Unbundle By Name(w189) -> ("window"=w182:dbl, "center"=w188:dbl)
        n74 = Not A Number/Path/Refnum?(number/path/refnum=w182) -> (NaN/Path/Refnum?=w185:bool)
        n75 = Not A Number/Path/Refnum?(number/path/refnum=w188) -> (NaN/Path/Refnum?=w184:bool)
        n76 = Or(x=w185, y=w184) -> (x .or. y?=w183:bool)
        n77 = case shown="False" w183 {
          tunnel: [w200 w201] -> w191
          tunnel: w190 -> [w199 w201]
          tunnel: w187 -> [w196 w202]
          tunnel: w188 -> [w195 _]
          tunnel: [w194 w202] -> w186
          tunnel: w182 -> [w193 _]
          frame False {
            w197 = T3[] [enum."-change center", enum."-write all X"] items=["balance", "h. offset change", "cursor moves", "change center", "change window", "init", "check", "reset", "set y to middle", "idle", "-write all Y", "-write left.X", "-write center.X", "-write right.X", "-write all X", "-change center", "-change window", "-change skew", "-read cursor 2", "-read cursor 1", "-read cursor 0", "-read all cursors", "-reset", "-read plot scale", "-set y to middle", "-Q: center.Y is visible", "-Q: window is visible", "-parse center.Y", "-right left from center", "-left move", "-right move", "-set center.Y", "-empty", "-set cursors to default", "-check", "-write center.Y", "-copy cursor 1", "-copy cursor 0", "-copy cursor 2", "move right", "move left", "shrink", "broaden", "skew up", "skew down", "-write plot scale", "zoom X", "change cen&win", "zoom to all data", "color--red", "color--green", "color--yellow", "read", "zoom out", "zoom in", "slide right", "slide left", "set range aspect ratio to 1", "move to window range", "--move to window range"]
            n78 = Bundle By Name(cluster=w196, "window"=w193, "center"=w195) -> (w194:T1)
            n79 = call "cursor window action stack.vi"("stack action"=stack_action_--_control."push", "action list"=w197, "command stack"=w199) -> ("command stack out"=w200:T3[])  [unwired: 6 in, 2 out]
          }
          frame True {
          }
        }
      }
      frame "change window" {
        n80 = Unbundle By Name(w207) -> ("window"=w205:dbl)
        n81 = Not A Number/Path/Refnum?(number/path/refnum=w205) -> (NaN/Path/Refnum?=w206:bool)
        n82 = case shown="False" w206 {
          tunnel: [w217 w218] -> w209
          tunnel: w208 -> [w216 w218]
          tunnel: w204 -> [w213 w219]
          tunnel: w205 -> [w212 _]
          tunnel: [w211 w219] -> w203
          frame False {
            w214 = T3[] [enum."-change window", enum."-write left.X", enum."-write right.X"] items=["balance", "h. offset change", "cursor moves", "change center", "change window", "init", "check", "reset", "set y to middle", "idle", "-write all Y", "-write left.X", "-write center.X", "-write right.X", "-write all X", "-change center", "-change window", "-change skew", "-read cursor 2", "-read cursor 1", "-read cursor 0", "-read all cursors", "-reset", "-read plot scale", "-set y to middle", "-Q: center.Y is visible", "-Q: window is visible", "-parse center.Y", "-right left from center", "-left move", "-right move", "-set center.Y", "-empty", "-set cursors to default", "-check", "-write center.Y", "-copy cursor 1", "-copy cursor 0", "-copy cursor 2", "move right", "move left", "shrink", "broaden", "skew up", "skew down", "-write plot scale", "zoom X", "change cen&win", "zoom to all data", "color--red", "color--green", "color--yellow", "read", "zoom out", "zoom in", "slide right", "slide left", "set range aspect ratio to 1", "move to window range", "--move to window range"]
            n83 = Bundle By Name(cluster=w213, "window"=w212) -> (w211:T1)
            n84 = call "cursor window action stack.vi"("stack action"=stack_action_--_control."push", "action list"=w214, "command stack"=w216) -> ("command stack out"=w217:T3[])  [unwired: 6 in, 2 out]
          }
          frame True {
          }
        }
      }
      frame "h. offset change" {
        n85 = Unbundle By Name(w224) -> ("h.offset"=w222:dbl)
        n86 = Not A Number/Path/Refnum?(number/path/refnum=w222) -> (NaN/Path/Refnum?=w223:bool)
        n87 = case shown="False" w223 {
          tunnel: [w234 w235] -> w226
          tunnel: w225 -> [w233 w235]
          tunnel: w221 -> [w230 w236]
          tunnel: w222 -> [w229 _]
          tunnel: [w228 w236] -> w220
          frame False {
            w231 = T3[] [enum."-change skew", enum."-write left.X", enum."-write right.X"] items=["balance", "h. offset change", "cursor moves", "change center", "change window", "init", "check", "reset", "set y to middle", "idle", "-write all Y", "-write left.X", "-write center.X", "-write right.X", "-write all X", "-change center", "-change window", "-change skew", "-read cursor 2", "-read cursor 1", "-read cursor 0", "-read all cursors", "-reset", "-read plot scale", "-set y to middle", "-Q: center.Y is visible", "-Q: window is visible", "-parse center.Y", "-right left from center", "-left move", "-right move", "-set center.Y", "-empty", "-set cursors to default", "-check", "-write center.Y", "-copy cursor 1", "-copy cursor 0", "-copy cursor 2", "move right", "move left", "shrink", "broaden", "skew up", "skew down", "-write plot scale", "zoom X", "change cen&win", "zoom to all data", "color--red", "color--green", "color--yellow", "read", "zoom out", "zoom in", "slide right", "slide left", "set range aspect ratio to 1", "move to window range", "--move to window range"]
            n88 = Bundle By Name(cluster=w230, "skew"=w229) -> (w228:T1)
            n89 = call "cursor window action stack.vi"("stack action"=stack_action_--_control."push", "action list"=w231, "command stack"=w233) -> ("command stack out"=w234:T3[])  [unwired: 6 in, 2 out]
          }
          frame True {
          }
        }
      }
      frame "reset" {
        w238 = T3[] [enum."-read plot scale", enum."-reset", enum."-write all X", enum."-write all Y"] items=["balance", "h. offset change", "cursor moves", "change center", "change window", "init", "check", "reset", "set y to middle", "idle", "-write all Y", "-write left.X", "-write center.X", "-write right.X", "-write all X", "-change center", "-change window", "-change skew", "-read cursor 2", "-read cursor 1", "-read cursor 0", "-read all cursors", "-reset", "-read plot scale", "-set y to middle", "-Q: center.Y is visible", "-Q: window is visible", "-parse center.Y", "-right left from center", "-left move", "-right move", "-set center.Y", "-empty", "-set cursors to default", "-check", "-write center.Y", "-copy cursor 1", "-copy cursor 0", "-copy cursor 2", "move right", "move left", "shrink", "broaden", "skew up", "skew down", "-write plot scale", "zoom X", "change cen&win", "zoom to all data", "color--red", "color--green", "color--yellow", "read", "zoom out", "zoom in", "slide right", "slide left", "set range aspect ratio to 1", "move to window range", "--move to window range"]
        n90 = call "cursor window action stack.vi"("stack action"=stack_action_--_control."push", "action list"=w238, "command stack"=w241) -> ("command stack out"=w240:T3[])  [unwired: 6 in, 2 out]
      }
      frame "set y to middle" {
        w245 = T3[] [enum."-read plot scale", enum."-set y to middle", enum."-write all Y"] items=["balance", "h. offset change", "cursor moves", "change center", "change window", "init", "check", "reset", "set y to middle", "idle", "-write all Y", "-write left.X", "-write center.X", "-write right.X", "-write all X", "-change center", "-change window", "-change skew", "-read cursor 2", "-read cursor 1", "-read cursor 0", "-read all cursors", "-reset", "-read plot scale", "-set y to middle", "-Q: center.Y is visible", "-Q: window is visible", "-parse center.Y", "-right left from center", "-left move", "-right move", "-set center.Y", "-empty", "-set cursors to default", "-check", "-write center.Y", "-copy cursor 1", "-copy cursor 0", "-copy cursor 2", "move right", "move left", "shrink", "broaden", "skew up", "skew down", "-write plot scale", "zoom X", "change cen&win", "zoom to all data", "color--red", "color--green", "color--yellow", "read", "zoom out", "zoom in", "slide right", "slide left", "set range aspect ratio to 1", "move to window range", "--move to window range"]
        n91 = call "cursor window action stack.vi"("stack action"=stack_action_--_control."push", "action list"=w245, "command stack"=w248) -> ("command stack out"=w247:T3[])  [unwired: 6 in, 2 out]
      }
      frame "-left move" {
        n92 = Unbundle By Name(w261) -> ("center"=w254:dbl, "skew.left"=w257:dbl, "skew.right"=w256:dbl)
        n93 = Unbundle By Name(w259) -> ("left.X"=w255:dbl)
        n94 = call "Q -- check range -- i -- real.vi"("upper"=w254, "number"=w255) -> ("selector"=w253:T2)  [unwired: 7 in, 2 out]
        n95 = case shown="\"in range\", Default" w253 {
          tunnel: w255 -> [w266 w284]
          tunnel: w256 -> [w272 w283]
          tunnel: [w273 w282] -> w262
          tunnel: [w268 w277] -> w264
          tunnel: w257 -> [w274 w281]
          tunnel: [w270 w276] -> w263
          tunnel: w254 -> [w267 w280]
          tunnel: [enum16{"forw", "back"}."forw" ("wing order") enum16{"forw", "back"}."back" ("wing order")] -> w252
          frame "in range", Default {
            # "right wing"
            # "left wing"
            n96 = Subtract(x=w267, y=w266) -> (x-y=w271:dbl)
            n97 = Divide(x=w271, y=w274) -> (x/y=w273:dbl)
            n98 = Multiply(x=w273, y=w272) -> (x*y=w269:dbl)
            n99 = Subtract(x=w267, y=w271) -> (x-y=w270:dbl)
            n100 = Add(x=w269, y=w267) -> (x+y=w268:dbl)
          }
          frame "above" {
            # "right wing"
            # "left wing"
            n101 = Subtract(x=w284, y=w280) -> (x-y=w279:dbl)
            n102 = Divide(x=w279, y=w283) -> (x/y=w282:dbl)
            n103 = Multiply(x=w282, y=w281) -> (x*y=w278:dbl)
            n104 = Subtract(x=w280, y=w278) -> (x-y=w276:dbl)
            n105 = Add(x=w279, y=w280) -> (x+y=w277:dbl)
          }
        }
        n106 = Bundle By Name(cluster=w261, "left"=w263, "right"=w264, "window"=w262, "wing order"=w252) -> (w251:T1)
      }
      frame "-right move" {
        n107 = Unbundle By Name(w295) -> ("center"=w286:dbl, "skew.left"=w291:dbl, "skew.right"=w290:dbl)
        n108 = Unbundle By Name(w293) -> ("right.X"=w289:dbl)
        n109 = call "Q -- check range -- i -- real.vi"("lower"=w286, "number"=w289) -> ("selector"=w288:T2)  [unwired: 7 in, 2 out]
        n110 = case shown="\"below\"" w288 {
          tunnel: w289 -> [w308 w310]
          tunnel: w290 -> [w307 w316]
          tunnel: [w306 w317] -> w296
          tunnel: [w301 w312] -> w298
          tunnel: w291 -> [w305 w318]
          tunnel: [w300 w314] -> w297
          tunnel: w286 -> [w304 w311]
          tunnel: [enum16{"forw", "back"}."forw" ("wing order") enum16{"forw", "back"}."back" ("wing order")] -> w287
          frame "in range", Default {
            # "right wing"
            n111 = Subtract(x=w308, y=w304) -> (x-y=w303:dbl)
            n112 = Divide(x=w303, y=w307) -> (x/y=w306:dbl)
            n113 = Multiply(x=w306, y=w305) -> (x*y=w302:dbl)
            n114 = Subtract(x=w304, y=w302) -> (x-y=w300:dbl)
            n115 = Add(x=w303, y=w304) -> (x+y=w301:dbl)
          }
          frame "below" {
            # "right wing"
            # "left wing"
            n116 = Subtract(x=w311, y=w310) -> (x-y=w315:dbl)
            n117 = Divide(x=w315, y=w318) -> (x/y=w317:dbl)
            n118 = Multiply(x=w317, y=w316) -> (x*y=w313:dbl)
            n119 = Subtract(x=w311, y=w315) -> (x-y=w314:dbl)
            n120 = Add(x=w313, y=w311) -> (x+y=w312:dbl)
          }
        }
        n121 = Bundle By Name(cluster=w295, "left"=w297, "right"=w298, "window"=w296, "wing order"=w287) -> (w285:T1)
      }
      frame "-set center.Y" {
        # "zero"
        # "calculate center.Y   from"
        # "complementary to calculation of fraction from vert offset"
        n122 = Unbundle By Name(w336) -> ("scale.y.halfwidth"=w333:dbl, "scale.y.center"=w334:dbl, "scale.x.range"=w340:dbl, "scale.y.max"=w339:dbl, "scale.y.min"=w338:dbl)
        n123 = Unbundle By Name(w330) -> ("window"=w341:dbl, "fixed vertical offset"=w342:dbl, "kind"=w320:enum16{"symmetric", "skewed", "fancy"}, "default window frac"=w343:dbl, "skew"=w319:dbl)
        n124 = case shown="\"symmetric\", Default" w320 {
          tunnel: w343 -> [w355 _]
          tunnel: w341 -> [w354 _]
          tunnel: w340 -> [w353 _]
          tunnel: [w344 w356] -> w321
          tunnel: w319 -> [_ w356]
          frame "symmetric", Default {
            # "window fraction"
            # "-1..1"
            n125 = Multiply(x=w353, y=w355) -> (x*y=w349:dbl)
            n126 = Divide(x=w354, y=w349) -> (x/y=w348:dbl)
            n127 = call "Q -- check range -- i -- real.vi"("upper"=0.99 ("y"), "lower"=0.0 ("y"), "number"=w348) -> ("number in range"=w345:dbl)  [unwired: 6 in, 2 out]
            n128 = Multiply(x=2.0, y=w345) -> (x*y=w352:dbl)
            n129 = Subtract(x=w352, y=1.0) -> (x-y=w344:dbl)
          }
          frame "skewed" {
          }
        }
        n130 = Multiply(x=w342, y=1.0) -> (x*y=w324:dbl)
        n131 = Multiply(x=w324, y=w333) -> (x*y=w329:dbl)
        n132 = Add(x=w334, y=w329) -> (x+y=w322:dbl)
        n133 = Subtract(x=w322, y=w338) -> (x-y=w327:dbl)
        n134 = Subtract(x=w339, y=w322) -> (x-y=w328:dbl)
        n135 = Max & Min(x=w328, y=w327) -> (min(x,y)=w326:dbl)  [unwired: 1 out]
        n136 = Multiply(x=w326, y=w321) -> (x*y=w323:dbl)
        n137 = Add(x=w322, y=w323) -> (x+y=w337:dbl)
        n138 = Bundle By Name(cluster=w336, "center.Y"=w337) -> (w335:T4)
      }
      frame "cursor moves" {
        n139 = Unbundle By Name(w369) -> ("cursors"=w368:i32[], "kind"=w359:enum16{"symmetric", "skewed", "fancy"})
        n140 = case shown="\"symmetric\", Default" w359 {
          tunnel: [w371 w375] -> w358
          tunnel: w357 -> [w371 w374]
          frame "symmetric", Default {
          }
          frame "fancy" {
            n141 = call "cursor window action stack.vi"("stack action"=stack_action_--_control."push", "cursor window action"=cursor_window_action."-write plot scale", "command stack"=w374) -> ("command stack out"=w375:T3[])  [unwired: 6 in, 2 out]
          }
        }
        n142 = Array Max & Min(array=w368) -> (max value=w366:i32, min value=w365:i32)  [unwired: 2 out]
        n143 = call "Q -- check range -- i -- integer.vi"("upper"=w366, "lower"=w365, "number"=w360) -> ("in range?"=w364:bool)  [unwired: 6 in, 2 out]
        n144 = Subtract(x=w360, y=w365) -> (x-y=w367:i32)
        n145 = case shown="True" w364 {
          tunnel: w358 -> [w377 w384]
          tunnel: [w377 w383] -> w370
          tunnel: w369 -> [w376 w382]
          tunnel: [w376 w381] -> w361
          tunnel: w368 -> [_ w380]
          tunnel: w367 -> [_ w379]
          frame False {
          }
          frame True {
            n146 = Index Array(array=w380, index=w379) -> (element=w378:i32)
            n147 = Bundle By Name(cluster=w382, "absolute"=w378, "relative"=w379) -> (w381:T1)
            n148 = case shown="0, 2, Default" w379 {
              selector: w379 -> [_ w394]
              tunnel: w384 -> [w388 w396]
              tunnel: [w387 w395] -> w383
              frame 1 {
                w385 = T3[] [enum."-read cursor 1", enum."-read plot scale", enum."-parse center.Y", enum."-copy cursor 1", enum."-change center", enum."-write right.X", enum."-write left.X"] items=["balance", "h. offset change", "cursor moves", "change center", "change window", "init", "check", "reset", "set y to middle", "idle", "-write all Y", "-write left.X", "-write center.X", "-write right.X", "-write all X", "-change center", "-change window", "-change skew", "-read cursor 2", "-read cursor 1", "-read cursor 0", "-read all cursors", "-reset", "-read plot scale", "-set y to middle", "-Q: center.Y is visible", "-Q: window is visible", "-parse center.Y", "-right left from center", "-left move", "-right move", "-set center.Y", "-empty", "-set cursors to default", "-check", "-write center.Y", "-copy cursor 1", "-copy cursor 0", "-copy cursor 2", "move right", "move left", "shrink", "broaden", "skew up", "skew down", "-write plot scale", "zoom X", "change cen&win", "zoom to all data", "color--red", "color--green", "color--yellow", "read", "zoom out", "zoom in", "slide right", "slide left", "set range aspect ratio to 1", "move to window range", "--move to window range"]
                n149 = call "cursor window action stack.vi"("stack action"=stack_action_--_control."push", "action list"=w385, "command stack"=w388) -> ("command stack out"=w387:T3[])  [unwired: 6 in, 2 out]
              }
              frame 0, 2, Default {
                w393 = T3[] [enum."-set center.Y", enum."-write center.Y"] items=["balance", "h. offset change", "cursor moves", "change center", "change window", "init", "check", "reset", "set y to middle", "idle", "-write all Y", "-write left.X", "-write center.X", "-write right.X", "-write all X", "-change center", "-change window", "-change skew", "-read cursor 2", "-read cursor 1", "-read cursor 0", "-read all cursors", "-reset", "-read plot scale", "-set y to middle", "-Q: center.Y is visible", "-Q: window is visible", "-parse center.Y", "-right left from center", "-left move", "-right move", "-set center.Y", "-empty", "-set cursors to default", "-check", "-write center.Y", "-copy cursor 1", "-copy cursor 0", "-copy cursor 2", "move right", "move left", "shrink", "broaden", "skew up", "skew down", "-write plot scale", "zoom X", "change cen&win", "zoom to all data", "color--red", "color--green", "color--yellow", "read", "zoom out", "zoom in", "slide right", "slide left", "set range aspect ratio to 1", "move to window range", "--move to window range"]
                w391 = T3[] [enum."-read plot scale"] items=["balance", "h. offset change", "cursor moves", "change center", "change window", "init", "check", "reset", "set y to middle", "idle", "-write all Y", "-write left.X", "-write center.X", "-write right.X", "-write all X", "-change center", "-change window", "-change skew", "-read cursor 2", "-read cursor 1", "-read cursor 0", "-read all cursors", "-reset", "-read plot scale", "-set y to middle", "-Q: center.Y is visible", "-Q: window is visible", "-parse center.Y", "-right left from center", "-left move", "-right move", "-set center.Y", "-empty", "-set cursors to default", "-check", "-write center.Y", "-copy cursor 1", "-copy cursor 0", "-copy cursor 2", "move right", "move left", "shrink", "broaden", "skew up", "skew down", "-write plot scale", "zoom X", "change cen&win", "zoom to all data", "color--red", "color--green", "color--yellow", "read", "zoom out", "zoom in", "slide right", "slide left", "set range aspect ratio to 1", "move to window range", "--move to window range"]
                n150 = case shown="0, Default" w394 {
                  tunnel: [w397 w398] -> w392
                  frame 0, Default {
                    w397 = T3[] [enum."-read cursor 0", enum."-left move", enum."-write right.X"] items=["balance", "h. offset change", "cursor moves", "change center", "change window", "init", "check", "reset", "set y to middle", "idle", "-write all Y", "-write left.X", "-write center.X", "-write right.X", "-write all X", "-change center", "-change window", "-change skew", "-read cursor 2", "-read cursor 1", "-read cursor 0", "-read all cursors", "-reset", "-read plot scale", "-set y to middle", "-Q: center.Y is visible", "-Q: window is visible", "-parse center.Y", "-right left from center", "-left move", "-right move", "-set center.Y", "-empty", "-set cursors to default", "-check", "-write center.Y", "-copy cursor 1", "-copy cursor 0", "-copy cursor 2", "move right", "move left", "shrink", "broaden", "skew up", "skew down", "-write plot scale", "zoom X", "change cen&win", "zoom to all data", "color--red", "color--green", "color--yellow", "read", "zoom out", "zoom in", "slide right", "slide left", "set range aspect ratio to 1", "move to window range", "--move to window range"]
                  }
                  frame 2 {
                    w398 = T3[] [enum."-read cursor 2", enum."-right move", enum."-write left.X"] items=["balance", "h. offset change", "cursor moves", "change center", "change window", "init", "check", "reset", "set y to middle", "idle", "-write all Y", "-write left.X", "-write center.X", "-write right.X", "-write all X", "-change center", "-change window", "-change skew", "-read cursor 2", "-read cursor 1", "-read cursor 0", "-read all cursors", "-reset", "-read plot scale", "-set y to middle", "-Q: center.Y is visible", "-Q: window is visible", "-parse center.Y", "-right left from center", "-left move", "-right move", "-set center.Y", "-empty", "-set cursors to default", "-check", "-write center.Y", "-copy cursor 1", "-copy cursor 0", "-copy cursor 2", "move right", "move left", "shrink", "broaden", "skew up", "skew down", "-write plot scale", "zoom X", "change cen&win", "zoom to all data", "color--red", "color--green", "color--yellow", "read", "zoom out", "zoom in", "slide right", "slide left", "set range aspect ratio to 1", "move to window range", "--move to window range"]
                  }
                }
                n151 = Build Array (concatenate)(w391, w392, w393) -> (w389:T3[])
                n152 = call "cursor window action stack.vi"("stack action"=stack_action_--_control."push", "action list"=w389, "command stack"=w396) -> ("command stack out"=w395:T3[])  [unwired: 6 in, 2 out]
              }
            }
          }
        }
      }
      frame "idle" {
      }
      frame "-copy cursor 1" {
        n153 = Unbundle By Name(w408) -> ("center.X"=w407:dbl)
        n154 = Bundle By Name(cluster=w405, "center"=w407) -> (w404:T1)
      }
      frame "-set y to middle" {
        w409 = 0.5
        n155 = Unbundle By Name(w412) -> ("fixed vertical offset"=w418:dbl)
        n156 = Unbundle By Name(w417) -> ("scale.y.center"=w413:dbl, "scale.y.halfwidth"=w414:dbl)
        n157 = Multiply(x=w414, y=w418) -> (x*y=w419:dbl)
        n158 = Bundle By Name(cluster=w412, "skew"=0.0, "skew.left"=w409, "skew.right"=w409) -> (w411:T1)
        n159 = Add(x=w413, y=w419) -> (x+y=w415:dbl)
        n160 = Bundle By Name(cluster=w417, "right.Y"=w415, "center.Y"=w415, "left.Y"=w415) -> (w416:T4)
      }
      frame "-set cursors to default" {
        w425 = 0.5
        w424 = 0.1
        (unwired) 3
        n161 = Unbundle By Name(w435) -> ("scale.x.halfwidth"=w423:dbl, "scale.x.center"=w429:dbl)
        n162 = Multiply(x=w423, y=w424) -> (x*y=w422:dbl)
        n163 = Multiply(x=w422, y=2) -> (x*y=w428:dbl)
        n164 = Add(x=w429, y=w422) -> (x+y=w433:dbl)
        n165 = Subtract(x=w429, y=w422) -> (x-y=w434:dbl)
        n166 = Bundle By Name(cluster=w431, "vertical offset"=0.0, "default window frac"=w424, "left"=w434, "right"=w433, "center"=w429, "window"=w428, "skew"=0.0, "skew.left"=w425, "skew.right"=w425) -> (w427:T1)
      }
      frame "-read plot scale" {
        w449 = 2.0 ("y")
        w454 = 2.0 ("y")
        n167 = Unbundle By Name(w445) -> ("Plot ref Syg"=w444:refnum<vi>)
        n168 = call "signal plot replace cursor - plot ref - V2.vi"("Signal graph IN"=w444, "cursor action"=cursor_action."check plot scale") -> ("2Dwindow bounds out"=w443:T10)  [unwired: 14 in, 3 out]
        n169 = Unbundle By Name(w443) -> ("max y"=w442:dbl, "min y"=w441:dbl, "max x"=w440:dbl, "min x"=w439:dbl)
        n170 = Add(x=w440, y=w439) -> (x+y=w455:dbl)
        n171 = Subtract(x=w440, y=w439) -> (x-y=w453:dbl)
        n172 = Divide(x=w455, y=w454) -> (x/y=w452:dbl)
        n173 = Divide(x=w453, y=w454) -> (x/y=w451:dbl)
        n174 = Subtract(x=w442, y=w441) -> (x-y=w446:dbl)
        n175 = Add(x=w442, y=w441) -> (x+y=w450:dbl)
        n176 = Divide(x=w450, y=w449) -> (x/y=w448:dbl)
        n177 = Divide(x=w446, y=w449) -> (x/y=w447:dbl)
        n178 = Bundle By Name(cluster=w458, "scale.y.max"=w442, "scale.y.min"=w441, "scale.x.max"=w440, "scale.x.min"=w439, "scale.x.range"=w453, "scale.x.halfwidth"=w451, "scale.x.center"=w452, "scale.y.range"=w446, "scale.y.halfwidth"=w447, "scale.y.center"=w448) -> (w457:T4)
      }
      frame "-write plot scale" {
        n179 = Unbundle By Name(w471) -> ("Plot ref Syg"=w464:refnum<vi>, "window"=w468:dbl, "center"=w467:dbl, "default window frac"=w466:dbl)
        n180 = call "Q -- range multiplier -- real -- V2.vi"("factor"=w466, "rage multiplier action"=range_multiplier_action."zoom", "center"=w467, "window"=w468) -> ("center OUT"=w462:dbl, "window OUT"=w461:dbl)  [unwired: 4 in, 2 out]
        n181 = Bundle By Name(cluster=T8 {"window y"=0.0021014740628288917, "center x"=44850.89441339177, "center y"=2.5658109925320947, "window x"=17480.201988350764} ("window IN"), "window x"=w461, "center x"=w462) -> (w460:T8)
        n182 = call "signal plot replace cursor - plot ref - V2.vi"("Signal graph IN"=w464, "window IN"=w460, "cursor action"=cursor_action."zoom to X win") -> ()  [unwired: 13 in, 4 out]
      }
      frame "zoom X" {
        n183 = Unbundle By Name(w486) -> ("Plot ref Syg"=w478:refnum<vi>, "window"=w477:dbl, "center"=w476:dbl, "default window frac"=w475:dbl)
        n184 = Reciprocal(x=w475) -> (1/x=w474:dbl)
        n185 = call "Q -- range multiplier -- real -- V2.vi"("factor"=w474, "rage multiplier action"=range_multiplier_action."zoom", "center"=w476, "window"=w477) -> ("center OUT"=w481:dbl, "window OUT"=w480:dbl)  [unwired: 4 in, 2 out]
        n186 = Bundle By Name(cluster=T8 {"window y"=0.0021014740628288917, "center x"=44850.89441339177, "center y"=2.5658109925320947, "window x"=17480.201988350764} ("window IN"), "window x"=w480, "center x"=w481) -> (w479:T8)
        n187 = call "signal plot replace cursor - plot ref - V2.vi"("Signal graph IN"=w478, "window IN"=w479, "cursor action"=cursor_action."zoom to X win") -> ()  [unwired: 13 in, 4 out]
      }
      frame "zoom out" {
        (unwired) range_multiplier_action."zoom" ("rage multiplier action")
        n188 = Unbundle By Name(w492) -> ("Plot ref Syg"=w489:refnum<vi>)
        n189 = call "signal plot replace cursor - plot ref - V2.vi"("Signal graph IN"=w489, "cursor action"=cursor_action."zoom out X") -> ()  [unwired: 14 in, 4 out]
      }
      frame "set range aspect ratio to 1" {
        n190 = Unbundle By Name(w498) -> ("Plot ref Syg"=w496:refnum<vi>)
        n191 = call "signal plot replace cursor - plot ref - V2.vi"("Signal graph IN"=w496, "cursor action"=cursor_action."zoom to aspect ratio 1") -> ()  [unwired: 14 in, 4 out]
      }
      frame "zoom in" {
        n192 = Unbundle By Name(w504) -> ("Plot ref Syg"=w502:refnum<vi>)
        n193 = call "signal plot replace cursor - plot ref - V2.vi"("Signal graph IN"=w502, "cursor action"=cursor_action."zoom in X") -> ()  [unwired: 14 in, 4 out]
      }
      frame "slide right" {
        n194 = Unbundle By Name(w510) -> ("Plot ref Syg"=w508:refnum<vi>)
        n195 = call "signal plot replace cursor - plot ref - V2.vi"("Signal graph IN"=w508, "cursor action"=cursor_action."move range right 20%") -> ()  [unwired: 14 in, 4 out]
      }
      frame "slide left" {
        n196 = Unbundle By Name(w516) -> ("Plot ref Syg"=w514:refnum<vi>)
        n197 = call "signal plot replace cursor - plot ref - V2.vi"("Signal graph IN"=w514, "cursor action"=cursor_action."move range left 20%") -> ()  [unwired: 14 in, 4 out]
      }
      frame "-Q: center.Y is visible" {
        # "check if y is within y-scale bounds"
        n198 = Unbundle By Name(w525) -> ("center.Y"=w528:dbl, "scale.y.max"=w527:dbl, "scale.y.min"=w526:dbl, "scale.y.center"=w519:dbl)
        n199 = call "Q -- check range -- i -- real.vi"("upper"=w527, "lower"=w526, "number"=w528) -> ("in range?"=w520:bool)  [unwired: 6 in, 2 out]
        n200 = case shown="False" w520 {
          tunnel: w525 -> [w536 w538]
          tunnel: [w535 w538] -> w524
          tunnel: w522 -> [w533 w537]
          tunnel: [w531 w537] -> w521
          tunnel: w519 -> [w530 _]
          frame False {
            w534 = T3[] [enum."-parse center.Y", enum."-write center.Y"] items=["balance", "h. offset change", "cursor moves", "change center", "change window", "init", "check", "reset", "set y to middle", "idle", "-write all Y", "-write left.X", "-write center.X", "-write right.X", "-write all X", "-change center", "-change window", "-change skew", "-read cursor 2", "-read cursor 1", "-read cursor 0", "-read all cursors", "-reset", "-read plot scale", "-set y to middle", "-Q: center.Y is visible", "-Q: window is visible", "-parse center.Y", "-right left from center", "-left move", "-right move", "-set center.Y", "-empty", "-set cursors to default", "-check", "-write center.Y", "-copy cursor 1", "-copy cursor 0", "-copy cursor 2", "move right", "move left", "shrink", "broaden", "skew up", "skew down", "-write plot scale", "zoom X", "change cen&win", "zoom to all data", "color--red", "color--green", "color--yellow", "read", "zoom out", "zoom in", "slide right", "slide left", "set range aspect ratio to 1", "move to window range", "--move to window range"]
            n201 = Bundle By Name(cluster=w536, "center.Y"=w530) -> (w535:T4)
            n202 = call "cursor window action stack.vi"("stack action"=stack_action_--_control."push", "action list"=w534, "command stack"=w533) -> ("command stack out"=w531:T3[])  [unwired: 6 in, 2 out]
          }
          frame True {
          }
        }
      }
      frame "move left" {
        (unwired) 0.2
        w551 = T3[] [enum."-change center", enum."-write all X"] items=["balance", "h. offset change", "cursor moves", "change center", "change window", "init", "check", "reset", "set y to middle", "idle", "-write all Y", "-write left.X", "-write center.X", "-write right.X", "-write all X", "-change center", "-change window", "-change skew", "-read cursor 2", "-read cursor 1", "-read cursor 0", "-read all cursors", "-reset", "-read plot scale", "-set y to middle", "-Q: center.Y is visible", "-Q: window is visible", "-parse center.Y", "-right left from center", "-left move", "-right move", "-set center.Y", "-empty", "-set cursors to default", "-check", "-write center.Y", "-copy cursor 1", "-copy cursor 0", "-copy cursor 2", "move right", "move left", "shrink", "broaden", "skew up", "skew down", "-write plot scale", "zoom X", "change cen&win", "zoom to all data", "color--red", "color--green", "color--yellow", "read", "zoom out", "zoom in", "slide right", "slide left", "set range aspect ratio to 1", "move to window range", "--move to window range"]
        n203 = Unbundle By Name(w547) -> ("center"=w541:dbl, "window"=w540:dbl, "default window frac"=w539:dbl)  [unwired: 1 out]
        n204 = Multiply(x=w540, y=w539) -> (x*y=w542:dbl)
        n205 = Subtract(x=w541, y=w542) -> (x-y=w545:dbl)
        n206 = Bundle By Name(cluster=w547, "center"=w545) -> (w546:T1)
        n207 = call "cursor window action stack.vi"("stack action"=stack_action_--_control."push", "action list"=w551, "command stack"=w549) -> ("command stack out"=w548:T3[])  [unwired: 6 in, 2 out]
      }
      frame "move right" {
        (unwired) 0.2
        w564 = T3[] [enum."-change center", enum."-write all X"] items=["balance", "h. offset change", "cursor moves", "change center", "change window", "init", "check", "reset", "set y to middle", "idle", "-write all Y", "-write left.X", "-write center.X", "-write right.X", "-write all X", "-change center", "-change window", "-change skew", "-read cursor 2", "-read cursor 1", "-read cursor 0", "-read all cursors", "-reset", "-read plot scale", "-set y to middle", "-Q: center.Y is visible", "-Q: window is visible", "-parse center.Y", "-right left from center", "-left move", "-right move", "-set center.Y", "-empty", "-set cursors to default", "-check", "-write center.Y", "-copy cursor 1", "-copy cursor 0", "-copy cursor 2", "move right", "move left", "shrink", "broaden", "skew up", "skew down", "-write plot scale", "zoom X", "change cen&win", "zoom to all data", "color--red", "color--green", "color--yellow", "read", "zoom out", "zoom in", "slide right", "slide left", "set range aspect ratio to 1", "move to window range", "--move to window range"]
        n208 = Unbundle By Name(w553) -> ("center"=w556:dbl, "window"=w555:dbl, "default window frac"=w554:dbl)  [unwired: 1 out]
        n209 = Multiply(x=w555, y=w554) -> (x*y=w557:dbl)
        n210 = Add(x=w556, y=w557) -> (x+y=w558:dbl)
        n211 = Bundle By Name(cluster=w553, "center"=w558) -> (w552:T1)
        n212 = call "cursor window action stack.vi"("stack action"=stack_action_--_control."push", "action list"=w564, "command stack"=w562) -> ("command stack out"=w561:T3[])  [unwired: 6 in, 2 out]
      }
      frame "shrink" {
        (unwired) 0.3
        w577 = T3[] [enum."-change window", enum."-write all X", enum."-read plot scale", enum."-set center.Y", enum."-write center.Y"] items=["balance", "h. offset change", "cursor moves", "change center", "change window", "init", "check", "reset", "set y to middle", "idle", "-write all Y", "-write left.X", "-write center.X", "-write right.X", "-write all X", "-change center", "-change window", "-change skew", "-read cursor 2", "-read cursor 1", "-read cursor 0", "-read all cursors", "-reset", "-read plot scale", "-set y to middle", "-Q: center.Y is visible", "-Q: window is visible", "-parse center.Y", "-right left from center", "-left move", "-right move", "-set center.Y", "-empty", "-set cursors to default", "-check", "-write center.Y", "-copy cursor 1", "-copy cursor 0", "-copy cursor 2", "move right", "move left", "shrink", "broaden", "skew up", "skew down", "-write plot scale", "zoom X", "change cen&win", "zoom to all data", "color--red", "color--green", "color--yellow", "read", "zoom out", "zoom in", "slide right", "slide left", "set range aspect ratio to 1", "move to window range", "--move to window range"]
        n213 = Unbundle By Name(w573) -> ("window"=w568:dbl, "window"=w567:dbl, "default window frac"=w565:dbl)
        n214 = Multiply(x=w567, y=w565) -> (x*y=w566:dbl)
        n215 = Subtract(x=w568, y=w566) -> (x-y=w571:dbl)
        n216 = Bundle By Name(cluster=w573, "window"=w571) -> (w572:T1)
        n217 = call "cursor window action stack.vi"("stack action"=stack_action_--_control."push", "action list"=w577, "command stack"=w575) -> ("command stack out"=w574:T3[])  [unwired: 6 in, 2 out]
      }
      frame "broaden" {
        (unwired) 0.3
        w585 = T3[] [enum."-change window", enum."-write all X", enum."-read plot scale", enum."-set center.Y", enum."-write center.Y"] items=["balance", "h. offset change", "cursor moves", "change center", "change window", "init", "check", "reset", "set y to middle", "idle", "-write all Y", "-write left.X", "-write center.X", "-write right.X", "-write all X", "-change center", "-change window", "-change skew", "-read cursor 2", "-read cursor 1", "-read cursor 0", "-read all cursors", "-reset", "-read plot scale", "-set y to middle", "-Q: center.Y is visible", "-Q: window is visible", "-parse center.Y", "-right left from center", "-left move", "-right move", "-set center.Y", "-empty", "-set cursors to default", "-check", "-write center.Y", "-copy cursor 1", "-copy cursor 0", "-copy cursor 2", "move right", "move left", "shrink", "broaden", "skew up", "skew down", "-write plot scale", "zoom X", "change cen&win", "zoom to all data", "color--red", "color--green", "color--yellow", "read", "zoom out", "zoom in", "slide right", "slide left", "set range aspect ratio to 1", "move to window range", "--move to window range"]
        n218 = Unbundle By Name(w579) -> ("window"=w583:dbl, "window"=w582:dbl, "default window frac"=w580:dbl)
        n219 = Multiply(x=w582, y=w580) -> (x*y=w581:dbl)
        n220 = Add(x=w583, y=w581) -> (x+y=w584:dbl)
        n221 = Bundle By Name(cluster=w579, "window"=w584) -> (w578:T1)
        n222 = call "cursor window action stack.vi"("stack action"=stack_action_--_control."push", "action list"=w585, "command stack"=w589) -> ("command stack out"=w588:T3[])  [unwired: 6 in, 2 out]
      }
      frame "skew up" {
        n223 = Unbundle By Name(w592) -> ("kind"=w591:enum16{"symmetric", "skewed", "fancy"})
        n224 = case shown="\"skewed\"" w591 {
          tunnel: w597 -> [w599 w609]
          tunnel: [w599 w608] -> w596
          tunnel: [w598 w607] -> w595
          tunnel: w592 -> [w598 w605]
          frame "symmetric", Default {
          }
          frame "skewed" {
            w611 = T3[] [enum."-change skew", enum."-read plot scale", enum."-set center.Y", enum."-write right.X", enum."-write left.X", enum."-write center.Y"] items=["balance", "h. offset change", "cursor moves", "change center", "change window", "init", "check", "reset", "set y to middle", "idle", "-write all Y", "-write left.X", "-write center.X", "-write right.X", "-write all X", "-change center", "-change window", "-change skew", "-read cursor 2", "-read cursor 1", "-read cursor 0", "-read all cursors", "-reset", "-read plot scale", "-set y to middle", "-Q: center.Y is visible", "-Q: window is visible", "-parse center.Y", "-right left from center", "-left move", "-right move", "-set center.Y", "-empty", "-set cursors to default", "-check", "-write center.Y", "-copy cursor 1", "-copy cursor 0", "-copy cursor 2", "move right", "move left", "shrink", "broaden", "skew up", "skew down", "-write plot scale", "zoom X", "change cen&win", "zoom to all data", "color--red", "color--green", "color--yellow", "read", "zoom out", "zoom in", "slide right", "slide left", "set range aspect ratio to 1", "move to window range", "--move to window range"]
            n225 = Unbundle By Name(w605) -> ("skew"=w606:dbl)
            n226 = Add(x=0.1, y=w606) -> (x+y=w603:dbl)
            n227 = call "Q -- check range -- i -- real.vi"("upper"=1, "lower"=-1, "number"=w603) -> ("number in range"=w600:dbl)  [unwired: 6 in, 2 out]
            n228 = Bundle By Name(cluster=w605, "skew"=w600) -> (w607:T1)
            n229 = call "cursor window action stack.vi"("stack action"=stack_action_--_control."push", "action list"=w611, "command stack"=w609) -> ("command stack out"=w608:T3[])  [unwired: 6 in, 2 out]
          }
        }
      }
      frame "skew down" {
        n230 = Unbundle By Name(w613) -> ("kind"=w612:enum16{"symmetric", "skewed", "fancy"})
        n231 = case shown="\"skewed\"" w612 {
          tunnel: w618 -> [w620 w631]
          tunnel: [w620 w630] -> w617
          tunnel: [w619 w629] -> w616
          tunnel: w613 -> [w619 w628]
          frame "symmetric", Default {
          }
          frame "skewed" {
            w623 = T3[] [enum."-change skew", enum."-read plot scale", enum."-set center.Y", enum."-write right.X", enum."-write left.X", enum."-write center.Y"] items=["balance", "h. offset change", "cursor moves", "change center", "change window", "init", "check", "reset", "set y to middle", "idle", "-write all Y", "-write left.X", "-write center.X", "-write right.X", "-write all X", "-change center", "-change window", "-change skew", "-read cursor 2", "-read cursor 1", "-read cursor 0", "-read all cursors", "-reset", "-read plot scale", "-set y to middle", "-Q: center.Y is visible", "-Q: window is visible", "-parse center.Y", "-right left from center", "-left move", "-right move", "-set center.Y", "-empty", "-set cursors to default", "-check", "-write center.Y", "-copy cursor 1", "-copy cursor 0", "-copy cursor 2", "move right", "move left", "shrink", "broaden", "skew up", "skew down", "-write plot scale", "zoom X", "change cen&win", "zoom to all data", "color--red", "color--green", "color--yellow", "read", "zoom out", "zoom in", "slide right", "slide left", "set range aspect ratio to 1", "move to window range", "--move to window range"]
            n232 = Unbundle By Name(w628) -> ("skew"=w622:dbl)
            n233 = Subtract(x=w622, y=0.1) -> (x-y=w627:dbl)
            n234 = call "Q -- check range -- i -- real.vi"("upper"=1, "lower"=-1, "number"=w627) -> ("number in range"=w624:dbl)  [unwired: 6 in, 2 out]
            n235 = Bundle By Name(cluster=w628, "skew"=w624) -> (w629:T1)
            n236 = call "cursor window action stack.vi"("stack action"=stack_action_--_control."push", "action list"=w623, "command stack"=w631) -> ("command stack out"=w630:T3[])  [unwired: 6 in, 2 out]
          }
        }
      }
      frame "-parse center.Y" {
        w645 = 1.0  # y
        w647 = 2.0  # y
        # "left factor"
        # "right factor"
        # "0 .. 1"
        # "-1 .. 1"
        # "-1..1"
        # "\"zero\""
        # "calculate horizontal offset and/or window \nfrom vertical position of center cursor"
        n237 = Unbundle By Name(w656) -> ("center.Y"=w641:dbl, "scale.y.max"=w639:dbl, "scale.y.min"=w640:dbl, "scale.y.center"=w637:dbl, "scale.y.halfwidth"=w649:dbl)
        n238 = Unbundle By Name(w652) -> ("fixed vertical offset"=w669:dbl)
        n239 = Multiply(x=w649, y=w669) -> (x*y=w667:dbl)
        n240 = call "Q -- check range -- i -- real.vi"("upper"=w639, "lower"=w640, "default"=w637, "number"=w641) -> ("number in range"=w638:dbl)  [unwired: 5 in, 2 out]
        n241 = Add(x=w667, y=w637) -> (x+y=w664:dbl)
        n242 = Unbundle By Name(w652) -> ("default window frac"=w657:dbl, "kind"=w658:enum16{"symmetric", "skewed", "fancy"}, "skew"=w654:dbl, "window"=w653:dbl)
        n243 = Unbundle By Name(w656) -> ("scale.x.range"=w655:dbl)
        n244 = Subtract(x=w664, y=w640) -> (x-y=w665:dbl)
        n245 = Subtract(x=w639, y=w664) -> (x-y=w666:dbl)
        n246 = Max & Min(x=w666, y=w665) -> (min(x,y)=w662:dbl)  [unwired: 1 out]
        n247 = Subtract(x=w638, y=w664) -> (x-y=w663:dbl)
        n248 = Divide(x=w663, y=w662) -> (x/y=w661:dbl)
        n249 = Multiply(x=w661, y=0.99) -> (x*y=w636:dbl)
        n250 = call "Q -- check range -- i -- real.vi"("upper"=1, "lower"=-1, "number"=w636) -> ("number in range"=w633:dbl)  [unwired: 6 in, 2 out]
        n251 = Bundle By Name(cluster=w656, "center.Y"=w638) -> (w659:T4)
        n252 = case shown="\"symmetric\", Default" w658 {
          tunnel: [w670 w681] -> w644
          tunnel: w633 -> [w679 w681]
          tunnel: w657 -> [w678 _]
          tunnel: w655 -> [w677 _]
          tunnel: [w671 w680] -> w651
          tunnel: w654 -> [w670 _]
          tunnel: w653 -> [_ w680]
          frame "symmetric", Default {
            # "0 .. 1"
            # "-1 .. 1"
            n253 = Add(x=w679, y=1.0) -> (x+y=w675:dbl)
            n254 = Divide(x=w675, y=2.0) -> (x/y=w673:dbl)
            n255 = Multiply(x=w678, y=w673) -> (x*y=w672:dbl)
            n256 = Multiply(x=w672, y=w677) -> (x*y=w671:dbl)
          }
          frame "skewed" {
          }
        }
        n257 = Add(x=w644, y=w645) -> (x+y=w646:dbl)
        n258 = Divide(x=w646, y=w647) -> (x/y=w642:dbl)
        n259 = Subtract(x=w645, y=w642) -> (x-y=w643:dbl)
        n260 = Bundle By Name(cluster=w652, "skew"=w644, "window"=w651, "skew.left"=w643, "skew.right"=w642) -> (w648:T1)
      }
      frame "-Q: window is visible" {
        n261 = Unbundle By Name(w692) -> ("scale.x.min"=w684:dbl, "scale.x.max"=w683:dbl, "scale.x.center"=w687:dbl, "scale.x.range"=w682:dbl)  [unwired: 1 out]
        n262 = Unbundle By Name(w686) -> ("center"=w691:dbl)
        n263 = call "Q -- check range -- i -- real.vi"("upper"=w683, "lower"=w684, "number"=w691) -> ("selector"=w690:T2)  [unwired: 6 in, 2 out]
        "selector" <- w690
        n264 = case shown="\"in range\"" w690 {
          tunnel: w689 -> [w699 w724]
          tunnel: [w698 w722] -> w688
          tunnel: w686 -> [w697 w721]
          tunnel: w687 -> [_ w720]
          tunnel: [w695 w719] -> w685
          tunnel: w684 -> [w705 _]
          tunnel: w683 -> [w704 _]
          tunnel: w682 -> [w696 _]
          frame "in range" {
            n265 = Unbundle By Name(w697) -> ("left"=w707:dbl, "right"=w706:dbl)
            n266 = call "Q -- check range -- i -- real.vi"("upper"=w704, "lower"=w705, "number"=w707) -> ("in range?"=w703:bool)  [unwired: 6 in, 2 out]
            n267 = call "Q -- check range -- i -- real.vi"("upper"=w704, "lower"=w705, "number"=w706) -> ("in range?"=w702:bool)  [unwired: 6 in, 2 out]
            n268 = Not(x=w703) -> (.not. x?=w701:bool)
            n269 = Not(x=w702) -> (.not. x?=w700:bool)
            n270 = And(x=w701, y=w700) -> (x .and. y?=w694:bool)
            n271 = case shown="True" w694 {
              tunnel: w699 -> [w709 w716]
              tunnel: [w709 w715] -> w698
              tunnel: w697 -> [w708 w714]
              tunnel: w696 -> [_ w712]
              tunnel: [w708 w710] -> w695
              frame False {
              }
              frame True {
                w718 = T3[] [enum."-change window", enum."-write left.X", enum."-write right.X"] items=["balance", "h. offset change", "cursor moves", "change center", "change window", "init", "check", "reset", "set y to middle", "idle", "-write all Y", "-write left.X", "-write center.X", "-write right.X", "-write all X", "-change center", "-change window", "-change skew", "-read cursor 2", "-read cursor 1", "-read cursor 0", "-read all cursors", "-reset", "-read plot scale", "-set y to middle", "-Q: center.Y is visible", "-Q: window is visible", "-parse center.Y", "-right left from center", "-left move", "-right move", "-set center.Y", "-empty", "-set cursors to default", "-check", "-write center.Y", "-copy cursor 1", "-copy cursor 0", "-copy cursor 2", "move right", "move left", "shrink", "broaden", "skew up", "skew down", "-write plot scale", "zoom X", "change cen&win", "zoom to all data", "color--red", "color--green", "color--yellow", "read", "zoom out", "zoom in", "slide right", "slide left", "set range aspect ratio to 1", "move to window range", "--move to window range"]
                n272 = Unbundle By Name(w714) -> ("default window frac"=w713:dbl)
                n273 = Multiply(x=w713, y=w712) -> (x*y=w711:dbl)
                n274 = Bundle By Name(cluster=w714, "window"=w711) -> (w710:T1)
                n275 = call "cursor window action stack.vi"("stack action"=stack_action_--_control."push", "action list"=w718, "command stack"=w716) -> ("command stack out"=w715:T3[])  [unwired: 6 in, 2 out]
              }
            }
          }
          frame "not a number", "above", "below", Default {
            w725 = T3[] [enum."-change center", enum."-write all X", enum."-Q: window is visible"] items=["balance", "h. offset change", "cursor moves", "change center", "change window", "init", "check", "reset", "set y to middle", "idle", "-write all Y", "-write left.X", "-write center.X", "-write right.X", "-write all X", "-change center", "-change window", "-change skew", "-read cursor 2", "-read cursor 1", "-read cursor 0", "-read all cursors", "-reset", "-read plot scale", "-set y to middle", "-Q: center.Y is visible", "-Q: window is visible", "-parse center.Y", "-right left from center", "-left move", "-right move", "-set center.Y", "-empty", "-set cursors to default", "-check", "-write center.Y", "-copy cursor 1", "-copy cursor 0", "-copy cursor 2", "move right", "move left", "shrink", "broaden", "skew up", "skew down", "-write plot scale", "zoom X", "change cen&win", "zoom to all data", "color--red", "color--green", "color--yellow", "read", "zoom out", "zoom in", "slide right", "slide left", "set range aspect ratio to 1", "move to window range", "--move to window range"]
            n276 = Bundle By Name(cluster=w721, "center"=w720) -> (w719:T1)
            n277 = call "cursor window action stack.vi"("stack action"=stack_action_--_control."push", "action list"=w725, "command stack"=w724) -> ("command stack out"=w722:T3[])  [unwired: 6 in, 2 out]
          }
        }
      }
      frame "-write all X" {
        w742 = cursor_action."write"  # action
        n278 = Unbundle By Name(w726) -> ("Plot ref Syg"=w727:refnum<vi>, "cursors"=w740:i32[], "left"=w734:dbl, "center"=w733:dbl, "right"=w732:dbl)
        n279 = Index Array(array=w740, index #1=0 ("cursor index"), index #2=1 ("cursor index"), index #3=2 ("cursor index")) -> (element #1=w741:i32, element #2=w737:i32, element #3=w735:i32)
        n280 = call "signal plot replace cursor - plot ref - V2.vi"("Signal graph IN"=w727, "new X"=w734, "cursor index"=w741, "cursor action"=w742) -> ("Signal graph OUT"=w731:refnum<vi>)  [unwired: 12 in, 3 out]
        n281 = call "signal plot replace cursor - plot ref - V2.vi"("Signal graph IN"=w731, "new X"=w733, "cursor index"=w737, "cursor action"=w742) -> ("Signal graph OUT"=w730:refnum<vi>)  [unwired: 12 in, 3 out]
        n282 = call "signal plot replace cursor - plot ref - V2.vi"("Signal graph IN"=w730, "new X"=w732, "cursor index"=w735, "cursor action"=w742) -> ()  [unwired: 12 in, 4 out]
      }
      frame "color--red" {
        w744 = cursor_sate."colored" ("cursor state")
        w745 = u32 16728794 ("Color Box")
        w746 = cursor_action."write"  # action
        n283 = Unbundle By Name(w747) -> ("Plot ref Syg"=w748:refnum<vi>, "cursors"=w761:i32[], "left"=w755:dbl, "center"=w754:dbl, "right"=w753:dbl)
        n284 = Index Array(array=w761, index #1=0 ("cursor index"), index #2=1 ("cursor index"), index #3=2 ("cursor index")) -> (element #1=w762:i32, element #2=w758:i32, element #3=w756:i32)
        n285 = call "signal plot replace cursor - plot ref - V2.vi"("Signal graph IN"=w748, "new X"=w755, "cursor index"=w762, "cursor action"=w746, "Color Box"=w745, "cursor state"=w744) -> ("Signal graph OUT"=w752:refnum<vi>)  [unwired: 10 in, 3 out]
        n286 = call "signal plot replace cursor - plot ref - V2.vi"("Signal graph IN"=w752, "new X"=w754, "cursor index"=w758, "cursor action"=w746, "Color Box"=w745, "cursor state"=w744) -> ("Signal graph OUT"=w751:refnum<vi>)  [unwired: 10 in, 3 out]
        n287 = call "signal plot replace cursor - plot ref - V2.vi"("Signal graph IN"=w751, "new X"=w753, "cursor index"=w756, "cursor action"=w746, "Color Box"=w745, "cursor state"=w744) -> ()  [unwired: 10 in, 4 out]
      }
      frame "color--green" {
        w764 = cursor_sate."colored" ("cursor state")
        w765 = u32 4250624 ("Color Box")
        w766 = cursor_action."write"  # action
        n288 = Unbundle By Name(w767) -> ("Plot ref Syg"=w768:refnum<vi>, "cursors"=w781:i32[], "left"=w775:dbl, "center"=w774:dbl, "right"=w773:dbl)
        n289 = Index Array(array=w781, index #1=0 ("cursor index"), index #2=1 ("cursor index"), index #3=2 ("cursor index")) -> (element #1=w782:i32, element #2=w778:i32, element #3=w776:i32)
        n290 = call "signal plot replace cursor - plot ref - V2.vi"("Signal graph IN"=w768, "new X"=w775, "cursor index"=w782, "cursor action"=w766, "Color Box"=w765, "cursor state"=w764) -> ("Signal graph OUT"=w772:refnum<vi>)  [unwired: 10 in, 3 out]
        n291 = call "signal plot replace cursor - plot ref - V2.vi"("Signal graph IN"=w772, "new X"=w774, "cursor index"=w778, "cursor action"=w766, "Color Box"=w765, "cursor state"=w764) -> ("Signal graph OUT"=w771:refnum<vi>)  [unwired: 10 in, 3 out]
        n292 = call "signal plot replace cursor - plot ref - V2.vi"("Signal graph IN"=w771, "new X"=w773, "cursor index"=w776, "cursor action"=w766, "Color Box"=w765, "cursor state"=w764) -> ()  [unwired: 10 in, 4 out]
      }
      frame "color--yellow" {
        w784 = cursor_sate."colored" ("cursor state")
        w785 = u32 16773632 ("Color Box")
        w786 = cursor_action."write"  # action
        n293 = Unbundle By Name(w787) -> ("Plot ref Syg"=w788:refnum<vi>, "cursors"=w801:i32[], "left"=w795:dbl, "center"=w794:dbl, "right"=w793:dbl)
        n294 = Index Array(array=w801, index #1=0 ("cursor index"), index #2=1 ("cursor index"), index #3=2 ("cursor index")) -> (element #1=w802:i32, element #2=w798:i32, element #3=w796:i32)
        n295 = call "signal plot replace cursor - plot ref - V2.vi"("Signal graph IN"=w788, "new X"=w795, "cursor index"=w802, "cursor action"=w786, "Color Box"=w785, "cursor state"=w784) -> ("Signal graph OUT"=w792:refnum<vi>)  [unwired: 10 in, 3 out]
        n296 = call "signal plot replace cursor - plot ref - V2.vi"("Signal graph IN"=w792, "new X"=w794, "cursor index"=w798, "cursor action"=w786, "Color Box"=w785, "cursor state"=w784) -> ("Signal graph OUT"=w791:refnum<vi>)  [unwired: 10 in, 3 out]
        n297 = call "signal plot replace cursor - plot ref - V2.vi"("Signal graph IN"=w791, "new X"=w793, "cursor index"=w796, "cursor action"=w786, "Color Box"=w785, "cursor state"=w784) -> ()  [unwired: 10 in, 4 out]
      }
      frame "-write all Y" {
        w820 = cursor_action."write"  # action
        n298 = Unbundle By Name(w808) -> ("Plot ref Syg"=w809:refnum<vi>, "cursors"=w818:i32[])
        n299 = Unbundle By Name(w807) -> ("left.Y"=w806:dbl, "center.Y"=w805:dbl, "right.Y"=w804:dbl)
        n300 = Index Array(array=w818, index #1=0 ("cursor index"), index #2=1 ("cursor index"), index #3=2 ("cursor index")) -> (element #1=w819:i32, element #2=w815:i32, element #3=w813:i32)
        n301 = call "signal plot replace cursor - plot ref - V2.vi"("Signal graph IN"=w809, "new  Y"=w806, "cursor index"=w819, "cursor action"=w820) -> ("Signal graph OUT"=w812:refnum<vi>)  [unwired: 12 in, 3 out]
        n302 = call "signal plot replace cursor - plot ref - V2.vi"("Signal graph IN"=w812, "new  Y"=w805, "cursor index"=w815, "cursor action"=w820) -> ("Signal graph OUT"=w811:refnum<vi>)  [unwired: 12 in, 3 out]
        n303 = call "signal plot replace cursor - plot ref - V2.vi"("Signal graph IN"=w811, "new  Y"=w804, "cursor index"=w813, "cursor action"=w820) -> ()  [unwired: 12 in, 4 out]
      }
      frame "-write left.X" {
        w835 = cursor_action."write"  # action
        n304 = Unbundle By Name(w822) -> ("Plot ref Syg"=w827:refnum<vi>, "cursors"=w833:i32[], "left"=w823:dbl, "right"=w824:dbl, "wing order"=w826:enum16{"forw", "back"})
        n305 = Index Array(array=w833, index #1=0 ("cursor index"), index #2=1 ("cursor index"), index #3=2 ("cursor index")) -> (element #1=w834:i32)  [unwired: 2 out]
        n306 = case shown="\"back\"" w826 {
          tunnel: [w837 w838] -> w825
          tunnel: w824 -> [_ w838]
          tunnel: w823 -> [w837 _]
          frame "forw", Default {
          }
          frame "back" {
          }
        }
        n307 = call "signal plot replace cursor - plot ref - V2.vi"("Signal graph IN"=w827, "new X"=w825, "cursor index"=w834, "cursor action"=w835) -> ()  [unwired: 12 in, 4 out]
      }
      frame "-write right.X" {
        w852 = cursor_action."write"  # action
        n308 = Unbundle By Name(w839) -> ("Plot ref Syg"=w845:refnum<vi>, "cursors"=w851:i32[], "left"=w841:dbl, "right"=w842:dbl, "wing order"=w844:enum16{"forw", "back"})
        n309 = Index Array(array=w851, index #1=0 ("cursor index"), index #2=1 ("cursor index"), index #3=2 ("cursor index")) -> (element #3=w840:i32)  [unwired: 2 out]
        n310 = case shown="\"back\"" w844 {
          tunnel: [w854 w855] -> w843
          tunnel: w842 -> [w854 _]
          tunnel: w841 -> [_ w855]
          frame "forw", Default {
          }
          frame "back" {
          }
        }
        n311 = call "signal plot replace cursor - plot ref - V2.vi"("Signal graph IN"=w845, "new X"=w843, "cursor index"=w840, "cursor action"=w852) -> ()  [unwired: 12 in, 4 out]
      }
      frame "-write center.X" {
        w866 = cursor_action."write"  # action
        n312 = Unbundle By Name(w858) -> ("Plot ref Syg"=w859:refnum<vi>, "cursors"=w865:i32[], "center"=w856:dbl)
        n313 = Index Array(array=w865, index #1=0 ("cursor index"), index #2=1 ("cursor index"), index #3=2 ("cursor index")) -> (element #2=w857:i32)  [unwired: 2 out]
        n314 = call "signal plot replace cursor - plot ref - V2.vi"("Signal graph IN"=w859, "new X"=w856, "cursor index"=w857, "cursor action"=w866) -> ()  [unwired: 12 in, 4 out]
      }
      frame "-write center.Y" {
        w878 = cursor_action."write"  # action
        n315 = Unbundle By Name(w871) -> ("Plot ref Syg"=w872:refnum<vi>, "cursors"=w877:i32[])
        n316 = Index Array(array=w877, index #1=0 ("cursor index"), index #2=1 ("cursor index"), index #3=2 ("cursor index")) -> (element #2=w868:i32)  [unwired: 2 out]
        n317 = Unbundle By Name(w870) -> ("center.Y"=w869:dbl)
        n318 = call "signal plot replace cursor - plot ref - V2.vi"("Signal graph IN"=w872, "new  Y"=w869, "cursor index"=w868, "cursor action"=w878) -> ()  [unwired: 12 in, 4 out]
      }
      frame "-read all cursors" {
        w900 = cursor_action."read"  # action
        n319 = Unbundle By Name(w880) -> ("Plot ref Syg"=w881:refnum<vi>, "cursors"=w898:i32[])
        n320 = Index Array(array=w898, index #1=0 ("cursor index"), index #2=1 ("cursor index"), index #3=2 ("cursor index")) -> (element #1=w899:i32, element #2=w895:i32, element #3=w893:i32)
        n321 = call "signal plot replace cursor - plot ref - V2.vi"("Signal graph IN"=w881, "cursor index"=w899, "cursor action"=w900) -> ("Signal graph OUT"=w892:refnum<vi>, "read X"=w888:dbl, "read Y"=w887:dbl)  [unwired: 13 in, 1 out]
        n322 = call "signal plot replace cursor - plot ref - V2.vi"("Signal graph IN"=w892, "cursor index"=w895, "cursor action"=w900) -> ("Signal graph OUT"=w891:refnum<vi>, "read X"=w886:dbl, "read Y"=w885:dbl)  [unwired: 13 in, 1 out]
        n323 = call "signal plot replace cursor - plot ref - V2.vi"("Signal graph IN"=w891, "cursor index"=w893, "cursor action"=w900) -> ("read X"=w884:dbl, "read Y"=w883:dbl)  [unwired: 13 in, 2 out]
        n324 = Bundle By Name(cluster=w890, "left.X"=w888, "left.Y"=w887, "center.X"=w886, "center.Y"=w885, "right.X"=w884, "right.Y"=w883) -> (w889:T4)
      }
      frame "read" {
      }
      frame "-read cursor 2" {
        w918 = cursor_action."read"  # action
        n325 = Unbundle By Name(w907) -> ("Plot ref Syg"=w908:refnum<vi>, "cursors"=w917:i32[])
        n326 = Index Array(array=w917, index #1=0 ("cursor index"), index #2=1 ("cursor index"), index #3=2 ("cursor index")) -> (element #3=w906:i32)  [unwired: 2 out]
        n327 = call "signal plot replace cursor - plot ref - V2.vi"("Signal graph IN"=w908, "cursor index"=w906, "cursor action"=w918) -> ("read X"=w911:dbl, "read Y"=w910:dbl)  [unwired: 13 in, 2 out]
        n328 = Bundle By Name(cluster=w913, "right.X"=w911, "right.Y"=w910) -> (w912:T4)
      }
      frame "-read cursor 1" {
        w932 = cursor_action."read"  # action
        n329 = Unbundle By Name(w920) -> ("Plot ref Syg"=w922:refnum<vi>, "cursors"=w931:i32[])
        n330 = Index Array(array=w931, index #1=0 ("cursor index"), index #2=1 ("cursor index"), index #3=2 ("cursor index")) -> (element #2=w921:i32)  [unwired: 2 out]
        n331 = call "signal plot replace cursor - plot ref - V2.vi"("Signal graph IN"=w922, "cursor index"=w921, "cursor action"=w932) -> ("read X"=w925:dbl, "read Y"=w924:dbl)  [unwired: 13 in, 2 out]
        n332 = Bundle By Name(cluster=w927, "center.X"=w925, "center.Y"=w924) -> (w926:T4)
      }
      frame "-read cursor 0" {
        w946 = cursor_action."read"  # action
        n333 = Unbundle By Name(w934) -> ("Plot ref Syg"=w936:refnum<vi>, "cursors"=w945:i32[])
        n334 = Index Array(array=w945, index #1=0 ("cursor index"), index #2=1 ("cursor index"), index #3=2 ("cursor index")) -> (element #1=w935:i32)  [unwired: 2 out]
        n335 = call "signal plot replace cursor - plot ref - V2.vi"("Signal graph IN"=w936, "cursor index"=w935, "cursor action"=w946) -> ("read X"=w939:dbl, "read Y"=w938:dbl)  [unwired: 13 in, 2 out]
        n336 = Bundle By Name(cluster=w941, "left.X"=w939, "left.Y"=w938) -> (w940:T4)
      }
    }
    n337 = call "cursor window action stack.vi"("stack action"=stack_action_--_control."check", "command stack"=w28) -> ("stack is empty ?"=w26:bool, "command stack out"=w27:T3[])  [unwired: 7 in, 1 out]
  }
  "cursor window out" <- w11
  n338 = property class="Clust (strict)"(reference=w19, "Value"=w11) -> (reference out=→"cursor window OUT":refnum<vi>)  [unwired: 1 in, 1 out]
